vi "Multi_Run_Prog.vi"(0 "Command filename":path, 1 "Setup mode":T9(ring)) -> ()   [LabVIEW 2010]
uses:
  Anemometry Sub Vis/Gen Trav/Traverse_cluster.ctl
  Anemometry Sub Vis/Gen Trav/Spacing.ctl
  Anemometry Sub Vis/Controls/Multi_run_mode.ctl
  Anemometry Sub Vis/Gen Trav/Route mapping/Route_Display_Mode.ctl
  Anemometry Sub Vis/Controls/User_Specific_mode.ctl
  Anemometry Sub Vis/Controls/Multi_Run_Case.ctl
  Anemometry Sub Vis/Gen Trav/Multi_Run_Status.ctl
  Anemometry Sub Vis/Controls/Tunnel_Coordinates.ctl
  Anemometry Sub Vis/Controls/Post_Process.ctl
  ADAM Client/Sub VIs/ADAM Controls/Traverse_Level_State.ctl
  ADAM Client/Sub VIs/ADAM Controls/Tunnel_speed_mode.ctl
  Anemometry Sub Vis/Controls/Overhead.ctl
  ADAM Client/Sub VIs/ADAM Controls/Remember_value_mode.ctl
  Anemometry Sub Vis/Gen Trav/Trav_mode.ctl
  ADAM Client/Sub VIs/ADAM Controls/Client_Source_Status.ctl
  ADAM Client/Sub VIs/ADAM Controls/Update_scan_value.ctl
  Anemometry Sub Vis/File/Setup_Filetype.ctl
  Anemometry Sub Vis/Globals/Meas_global.vi
  Anemometry Sub Vis/Globals/Trav_pos_global.vi
  Anemometry Sub Vis/Globals/Preference_global.vi
  Anemometry Sub Vis/Gen Trav/Route mapping/Route_mapping_global.vi
  Anemometry Sub Vis/Globals/Extra_Commands_Global.vi
  Anemometry Sub Vis/Globals/LDA_meas_global_2.vi
  Anemometry Sub Vis/Globals/LDA_meas_global_1.vi
panel:
  out "Last Row Run":i32
  in  "Stop after Repeats":bool
  in  "Jump Bad Positions":bool
  in  "Work in Tunnel Coordinates?":T1
  out "Current Overhead Factor":dbl format="%.3f"
  out "Estimated Completion time":string
  out "Max Tunnel Speed":dbl format="%.2f"
  out "Pause message":string
  in  "Pause":bool
  out "Non Starter":bool
  out "No of Rows":i32
  out "Status":T2
  in  "Synchronization Start No":i32=1 min=1 max=100
  out "Multi Run Case":T3
  out "Simulate/Run":T4
  in  "Display Mode":T5=enum."Display View on Crash"
  in  "stop":bool
  out "Currently on Row":i32
  in  "Table":T6[](array[typedef]) {"Row Duration (mins)" format="%#.1f"; "Row No" min=0; "Trace Gas Concentration (%)" min=0.0 format="%#.2f"; "Emission Rate (l/min)" format="%#.2f"; "Tunnel Speed" format="%#.2f"; "Start X" format="%#.2f"; "Start Y" format="%#.2f"; "Start Z" format="%#.2f"; "End X" format="%#.2f"; "End Y" format="%#.2f"; "End Z" format="%#.2f"; "Averaging time (min)" min=0.0 format="%#.2f"}
  # "X           Y            Z"
  # "Start"
  # "End"
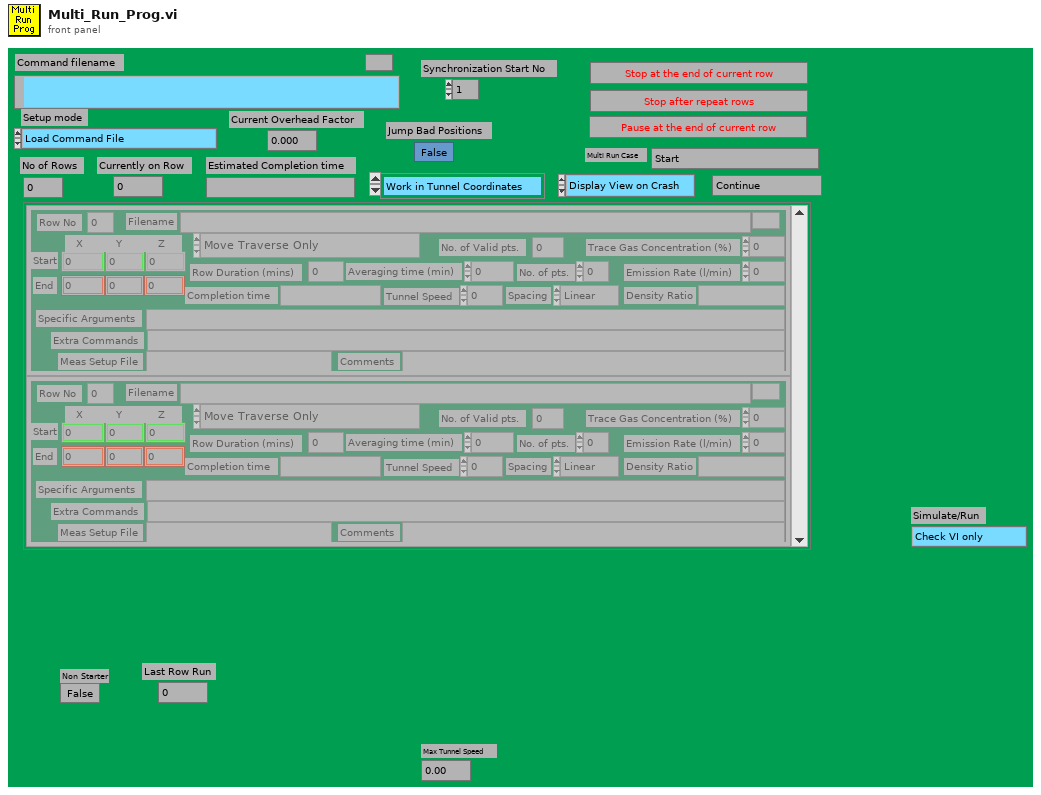
[diagram p1: front panel]
types:
  T1 = typedef "Tunnel_Coordinates.ctl" = enum16{"Work in Tunnel Coordinates", "Work in Model Coordinates"}
  T2 = typedef "Multi_Run_Status.ctl" = enum16{"Continue", "Jump to Next Point", "Jump to Next Row", "Jump To Fall Back", "Terminate Run"}
  T3 = typedef "Multi_Run_Case.ctl" = enum16{"Start", "Load Setup From File", "Has file been edited in Excel?", "Check Max Tunnel Speed", "Pre Check Row", "Check Rows", "Remove blank end rows", "Do results files already exist?", "FFID Bkgnd Measurements?", "First Save Setup file", "Setup Route checking", "Initialise Measurement Prog", "Input Current Position", "Experimental setup control", "Check source flowrates", "Setup for running mode", "Skip Blank Rows", "Which row to execute next", "Evaluate IF Statement", "Perform Measurement Setup", "Set Measurement Conditions", "Execute Row", "Calculate Row TIme", "Update time estimate", "Pause Multi Run Program", "Do Another Row?", "Find Next Fall Back Row", "Shut down source etc", "Email results to users", "Save run efficiency", "Remove Skipped Commands", "Show jumped positions", "Save Setup to File", "End"}
  T4 = typedef "User_Specific_mode.ctl" = enum16{"Check VI only", "Run VI"}
  T5 = typedef "Route_Display_Mode.ctl" = enum16{"Display View Always", "Display View on Crash"}
  T6 = typedef "Traverse_cluster.ctl" = cluster{"Start X":dbl, "Start Y":dbl, "Start Z":dbl, "End X":dbl, "End Y":dbl, "End Z":dbl, "No. of pts.":i32, "Spacing":T7, "Filename":path, "Tunnel Speed":dbl, "Averaging time (min)":dbl, "Extra Commands":string, "Specific Arguments":string, "Emission Rate (l/min)":dbl, "Trace Gas Concentration (%)":dbl, "Density Ratio":string, "Comments":string, "Row No":i32, "Row Type Selector":T8, "Completion time":string, "Row Duration (mins)":dbl, "No. of Valid pts.":i32, "Meas Setup File":string}
  T7 = typedef "Spacing.ctl" = enum16{"Linear", "Log", "Gauss", "Specified", "N/A"}
  T8 = typedef "Multi_run_mode.ctl" = enum16{"Move Traverse Only", "Set Tunnel Speed Only", "Set Source Only", "Set Measurement Conditions", "Single Measurement", "Vertical Profile", "Lateral Profile", "Longitudinal Profile", "Explore Volume", "Multi-Axis Profile", "Auto Calibrate", "Meas Fast FID Bkgnd", "Check Beam Power", "Scanning Valve Measurement", "Run VI Named:", "Set ADAM Ch", "Wait (minutes)", "Send Message", "Synchronize With:", "Fall Back to this Row", "Turn Off Row Repeating", "Blank Row"}
  T9 = enum16{"Load Command File", "Save Command File", "Check Multi Run Prog", "Check Multi Run Prog With Live Moves", "Run Multi Run Prog"}
  T10 = typedef "Post_Process.ctl" = enum16{"Take New Data", "Post Process Raw Data File"}
  T11 = typedef "Traverse_Level_State.ctl" = enum16{"Running", "Complete"}
  T12 = enum32{"existing file", "new file", "new or existing file", "existing dir", "new dir", "new or existing dir", "existing file (use LLBs)", "new file (use LLBs)", "new or existing file (use LLBs)", "new or existing file or directory (use LLBs)"}
  T13 = typedef "Tunnel_speed_mode.ctl" = enum16{"Set Speed", "Set Speed then wait", "Is tunnel speed allowable?"}
  T14 = enum16{"All Channel Names", "Valid Channel Names"}
  T15 = typedef "Overhead.ctl" = enum16{"Update total times", "Read Current Overhead", "Re Scale totals to 3 hrs", "Initialise totals to 3hr"}
  T16 = typedef "Remember_value_mode.ctl" = enum16{"Read only", "Read and Write"}
  T17 = typedef "Trav_mode.ctl" = enum16{"Move traverse", "Read traverse position", "Teach Position"}
  T18 = typedef "Client_Source_Status.ctl" = enum16{"Not Using", "Using", "Must Have"}
  T19 = typedef "Update_scan_value.ctl" = cluster{"Channel Name":string, "New Value":dbl}
  T20 = typedef "Setup_Filetype.ctl" = enum16{"Measurement Setups", "Calibration Setups", "General", "Results File Plotter Setups", "Speed Calib Tweaks"}
  T21 = enum16{"To Traverse Coordinates", "To User Coordinates"}
  T22 = typedef "Status_Cluster.ctl" = cluster{"Status":T2, "Error Type":string, "Error Description":string}
  T23 = typedef "BSA_info_Cluster.ctl" = cluster{"GPIB Address":string, "No of Check Bytes":i32, "Extra Info":string, "COLOUR":u32, "Wavelength (nm)":dbl}
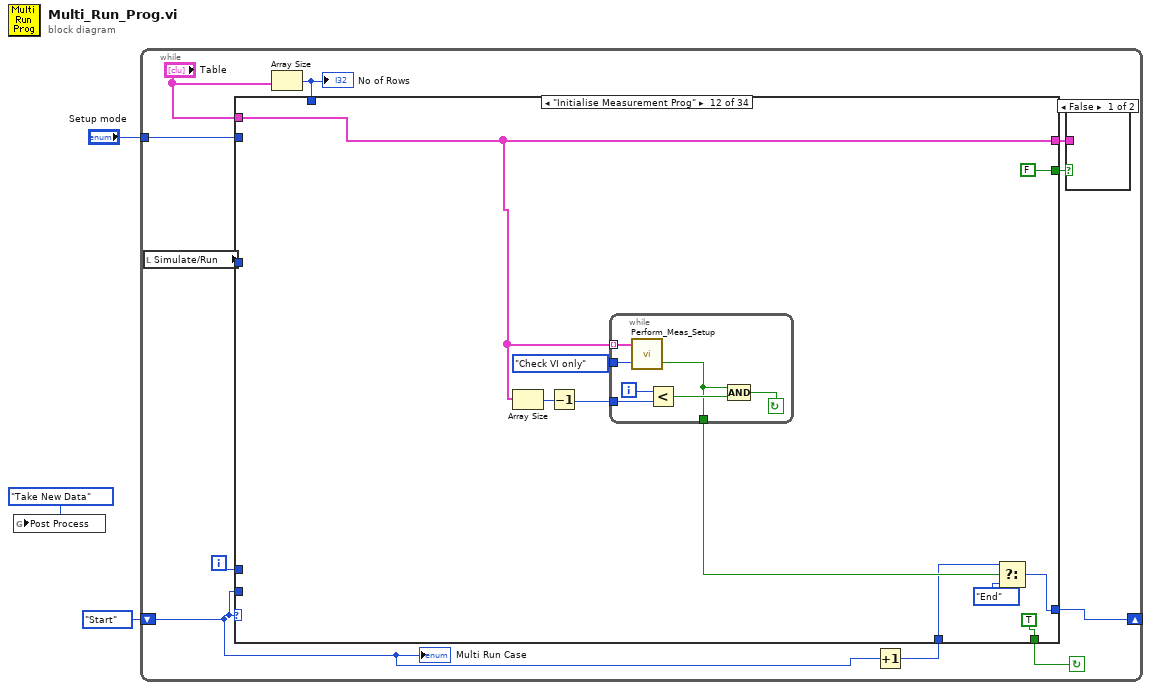
[diagram p0: block diagram]
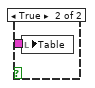
[diagram p2: hidden frame]
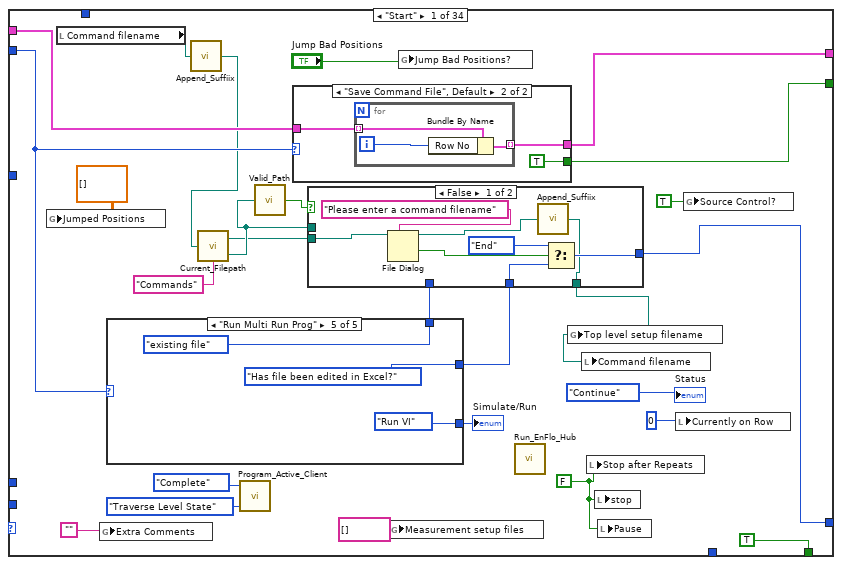
[diagram p3: hidden frame]
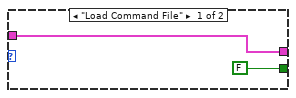
[diagram p4: hidden frame]
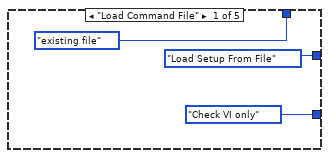
[diagram p6: hidden frame]
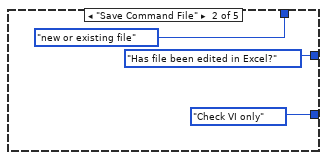
[diagram p7: hidden frame]
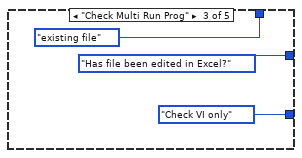
[diagram p8: hidden frame]
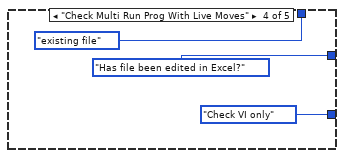
[diagram p9: hidden frame]
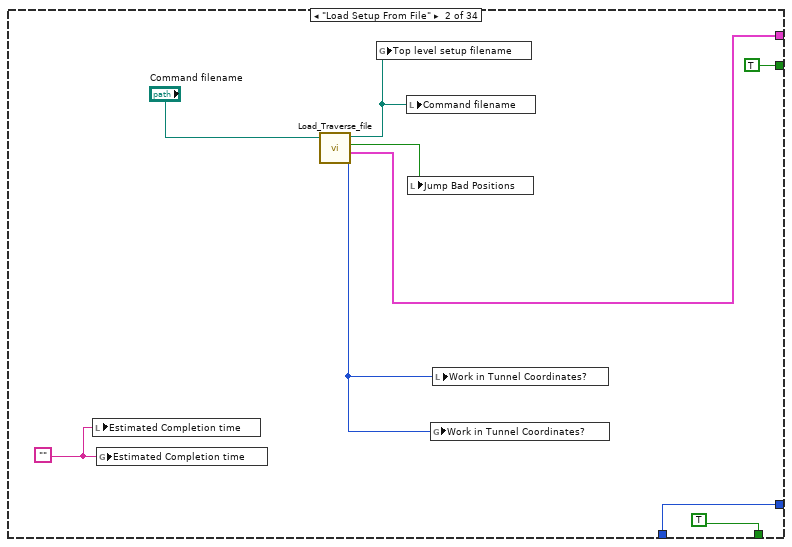
[diagram p10: hidden frame]
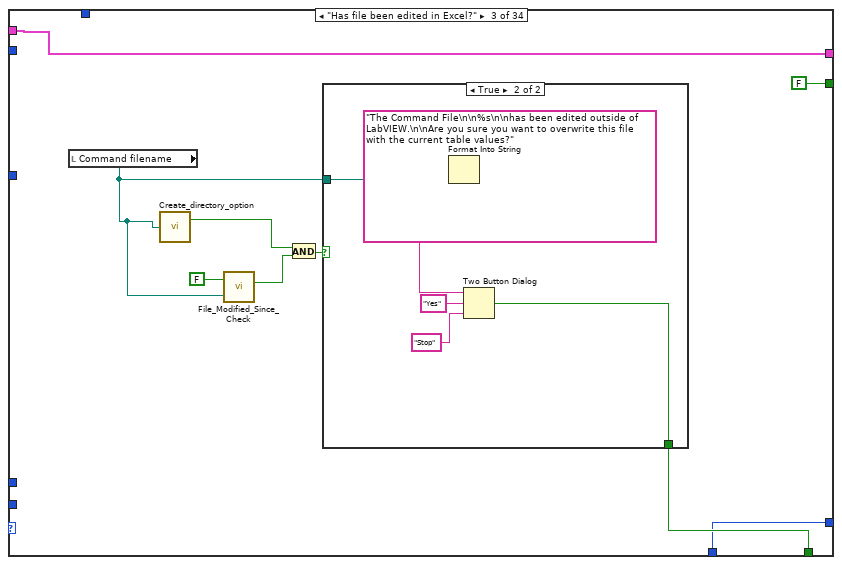
[diagram p11: hidden frame]
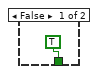
[diagram p12: hidden frame]
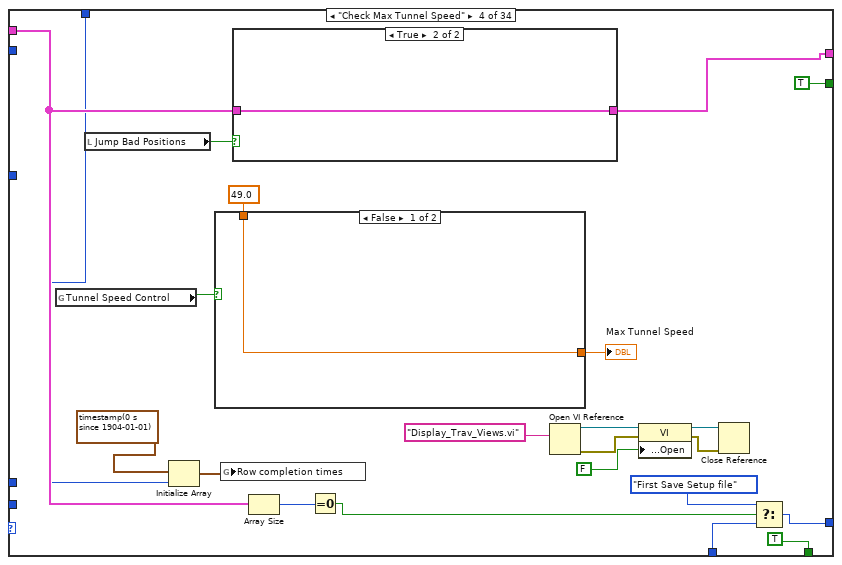
[diagram p13: hidden frame]
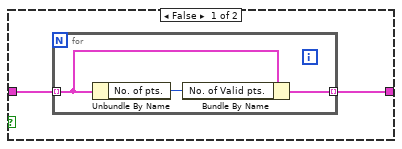
[diagram p14: hidden frame]
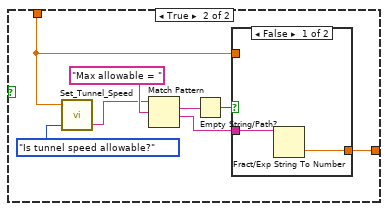
[diagram p15: hidden frame]
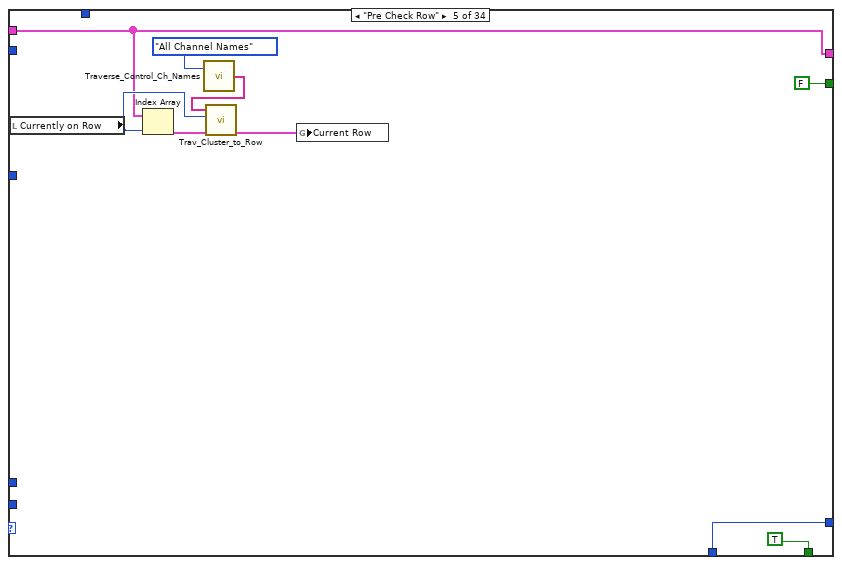
[diagram p17: hidden frame]
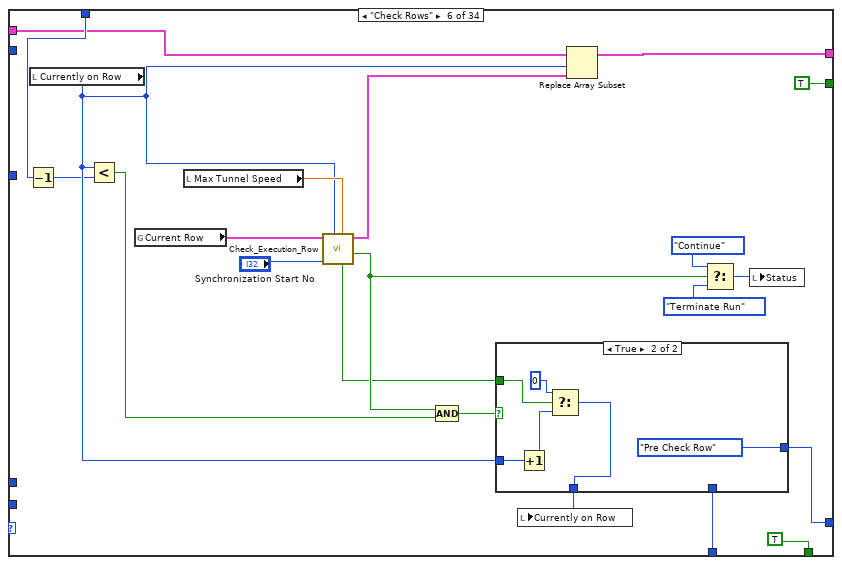
[diagram p18: hidden frame]
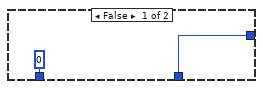
[diagram p19: hidden frame]
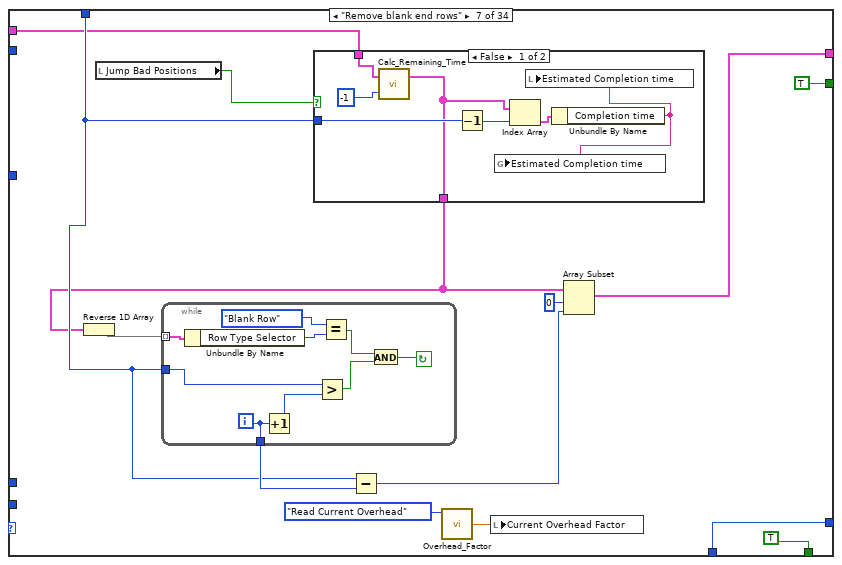
[diagram p20: hidden frame]
diagram:
  n1 = global write "Meas_global.vi" "Post Process"(Post_Process."Take New Data" ("Post Process")) -> ()
  n2 = while {
    shift-left: Multi_Run_Case."Start" ("Multi Run Case") -> [w10]
    shift-right: [w6] -> _
    tunnel: "Setup mode" -> [w13]
    i -> [w11]
    stop <- w14 continue-if-true
    n3 = local read "Simulate/Run"() -> (w7:T4)
    n4 = Array Size(array="Table") -> (size(s)=w5:i32)
    "No of Rows" <- w5
    n5 = Increment(x=w10) -> (x+1=w12:T3)
    n6 = case shown="\"Initialise Measurement Prog\"" w10 {
      tunnel: [TRUE TRUE w87 TRUE TRUE TRUE TRUE TRUE TRUE TRUE TRUE ("Continue?") TRUE ("Continue?") TRUE TRUE TRUE w520 TRUE ("Continue?") TRUE ("Continue?") TRUE TRUE ("Continue?") TRUE TRUE TRUE TRUE TRUE TRUE TRUE TRUE TRUE TRUE TRUE TRUE TRUE FALSE] -> w14
      tunnel: w13 -> [w26 _ _ _ _ _ _ _ _ w395 _ _ _ _ _ _ _ _ _ _ _ _ _ _ _ _ _ _ _ _ _ _ w1245 _]
      tunnel: "Table" -> [w39 _ w84 w114 w142 w154 w179 w210 w368 w397 w416 w456 w469 w497 w507 w523 w575 w619 w735 w786 w798 w889 w925 w957 w998 w1040 w1075 w1105 w1134 w1179 w1184 w1193 w1266 w1329]
      tunnel: w7 -> [_ _ _ _ _ _ _ w209 _ _ _ _ _ w501 w506 w522 _ w617 w732 w783 w796 w888 w923 w954 _ w1049 _ w1096 _ _ _ _ w1256 _]
      tunnel: w10 -> [_ _ _ _ _ _ _ _ _ _ _ _ _ _ _ _ _ _ _ _ _ _ _ _ _ _ _ _ _ _ _ _ _ _]
      tunnel: w12 -> [_ w80 w86 w112 w146 w156 w190 w214 w363 w394 w423 w453 w470 w496 w512 w525 w577 w615 w740 w787 w805 w886 w915 w959 w1001 _ _ w1089 w1136 w1181 w1187 w1201 w1264 w1328]
      tunnel: w11 -> [_ _ _ _ _ _ _ _ _ _ _ _ _ _ _ _ _ _ _ _ _ _ _ _ w999 _ _ _ _ _ _ _ _ _]
      tunnel: [w37 w80 w86 w111 w146 w155 w190 w214 w363 w390 w423 w452 w470 w496 w509 w525 w577 w616 w739 w787 w806 w886 w915 w959 w1002 w1050 w1072 w1100 w1136 w1181 w1187 w1201 w1264 w1328] -> w6
      tunnel: [w25 TRUE FALSE ("Rows Added ?") TRUE ("Rows Added ?") FALSE TRUE TRUE FALSE FALSE TRUE FALSE FALSE FALSE FALSE FALSE TRUE FALSE ("Rows Added ?") FALSE ("Rows Added ?") FALSE FALSE ("Rows Added ?") FALSE FALSE FALSE TRUE ("Rows Added ?") FALSE FALSE FALSE FALSE FALSE FALSE TRUE TRUE TRUE FALSE] -> w8
      tunnel: w5 -> [_ _ _ w106 _ w160 w181 _ _ _ _ _ _ _ _ _ w578 w618 _ _ _ _ _ w953 _ w1035 _ _ _ _ _ _ _ _]
      tunnel: [w38 w81 w84 w116 w142 w163 w185 w210 w368 w398 w416 w456 w469 w497 w507 w521 w575 w620 w735 w786 w798 w889 w925 w956 w998 w1040 w1075 w1105 w1134 w1179 w1183 w1193 w1265 w1329] -> w4
      frame "Start" {
        w23 = FALSE ("Measurment setup Found?")
        n7 = global write "Trav_pos_global.vi" "Jumped Positions"(dbl[][] [] ("Jumped Positions")) -> ()
        n8 = local read "Command filename"() -> (w29:path)
        n9 = global write "Meas_global.vi" "Extra Comments"("") -> ()
        n10 = case shown="\"Run Multi Run Prog\"" w26 {
          tunnel: [User_Specific_mode."Check VI only" ("Simulate/Run") User_Specific_mode."Check VI only" ("Simulate/Run") User_Specific_mode."Check VI only" ("Simulate/Run") User_Specific_mode."Check VI only" ("Simulate/Run") User_Specific_mode."Run VI" ("Simulate/Run")] -> w40
          tunnel: [Multi_Run_Case."Load Setup From File" ("Multi Run Case") Multi_Run_Case."Has file been edited in Excel?" ("Multi Run Case") Multi_Run_Case."Has file been edited in Excel?" ("Multi Run Case") Multi_Run_Case."Has file been edited in Excel?" ("Multi Run Case") Multi_Run_Case."Has file been edited in Excel?" ("Multi Run Case")] -> w36
          tunnel: [T12."existing file" ("select mode (2)") T12."new or existing file" ("select mode (2)") T12."existing file" ("select mode (2)") T12."existing file" ("select mode (2)") T12."existing file" ("select mode (2)")] -> w24
          frame "Load Command File" {
          }
          frame "Save Command File" {
          }
          frame "Check Multi Run Prog" {
          }
          frame "Check Multi Run Prog With Live Moves" {
          }
          frame "Run Multi Run Prog" {
          }
        }
        "Simulate/Run" <- w40
        n11 = call "Append_Suffiix.vi"("Results file"=w29) -> ("appended path"=w18:path)
        n12 = call "Current_Filepath.vi"("Filename in"=w18, "Data Type"="Commands") -> ("Filename Out"=w17:path, "Directory"=w16:path)
        n13 = call "Program_Active_Client.vi"("Mode"=enum16{"Program Active", "Traverse Level State"}."Traverse Level State", "Traverse level State"=Traverse_Level_State."Complete") -> ()  [unwired: 1 in, 3 out]
        n14 = call "Valid_Path.vi"("Filename"=w17) -> ("Valid Path?"=w27:bool)
        n15 = case shown="\"Save Command File\", Default" w26 {
          tunnel: w39 -> [w43 w46]
          tunnel: [w43 w45] -> w38
          tunnel: [FALSE TRUE] -> w25
          frame "Load Command File" {
          }
          frame "Save Command File", Default {
            n16 = for {
              tunnel: w46 -> [w49] mode=indexing
              tunnel: [w48] -> w45 mode=indexing
              i -> [w47]
              n17 = Bundle By Name(cluster=w49, "Row No"=w47) -> (w48:T6)
            }
          }
        }
        n18 = case shown="False" w27 {
          tunnel: [w55 w59] -> w37
          tunnel: w36 -> [w56 w59]
          tunnel: w17 -> [_ w58]
          tunnel: [w54 w58] -> w28
          tunnel: w24 -> [_ _]
          tunnel: w16 -> [w50 _]
          frame False {
            n19 = File Dialog(7:"Please enter a command filename" ("prompt"), 11:w50) -> (1:w52:bool, 3:w53:path)  [unwired: 1 in, 6 out]
            n20 = call "Append_Suffiix.vi"("Results file"=w53) -> ("appended path"=w54:path)
            n21 = Select(t=Multi_Run_Case."End" ("Multi Run Case"), s=w52, f=w56) -> (s? t:f=w55:T3)
          }
          frame True {
          }
        }
        n22 = global write "Trav_pos_global.vi" "Measurement setup files"(string[] [] ("Measurement setup files")) -> ()
        n23 = global write "Trav_pos_global.vi" "Jump Bad Positions?"("Jump Bad Positions") -> ()
        n24 = call "Run_EnFlo_Hub.vi"() -> ()  [unwired: 8 out]
        n25 = global write "Trav_pos_global.vi" "Top level setup filename"(w28) -> ()
        n26 = local write "Command filename"(w28) -> ()
        n27 = local write "Stop after Repeats"(w23) -> ()
        n28 = local write "stop"(w23) -> ()
        n29 = local write "Pause"(w23) -> ()
        n30 = local write "Currently on Row"(0 ("Currently on Row")) -> ()
        n31 = global write "Trav_pos_global.vi" "Source Control?"(TRUE ("Source Control?")) -> ()
        "Status" <- Multi_Run_Status."Continue" ("Status")
      }
      frame "Load Setup From File" {
        w76 = ""
        n32 = local write "Estimated Completion time"(w76) -> ()
        n33 = global write "Trav_pos_global.vi" "Estimated Completion time"(w76) -> ()
        n34 = call "Load_Traverse_file.vi"("Setup filename"="Command filename") -> ("Setup filename Out"=w78:path, "Jump Bad Positions"=w75:bool, "Table"=w81:T6[], "Work in Tunnel Coordinates?"=w77:T1)  [unwired: 2 out]
        n35 = global write "Trav_pos_global.vi" "Top level setup filename"(w78) -> ()
        n36 = local write "Command filename"(w78) -> ()
        n37 = local write "Jump Bad Positions"(w75) -> ()
        n38 = global write "Trav_pos_global.vi" "Work in Tunnel Coordinates?"(w77) -> ()
        n39 = local write "Work in Tunnel Coordinates?"(w77) -> ()
      }
      frame "Has file been edited in Excel?" {
        n40 = local read "Command filename"() -> (w88:path)
        n41 = call "Create_directory_option.vi"("Filename"=w88) -> ("Path is to existing File"=w91:bool)  [unwired: 1 out]
        n42 = call "File_Modified_Since_Check.vi"("Pathname"=w88, "Just Modified?"=FALSE) -> ("Modified?"=w90:bool)
        n43 = And(x=w91, y=w90) -> (x .and. y?=w92:bool)
        n44 = case shown="True" w92 {
          tunnel: w88 -> [_ w99]
          tunnel: [TRUE ("T button?") w94] -> w87
          frame False {
          }
          frame True {
            n45 = Format Into String(format string="The Command File\n\n%s\n\nhas been edited outside of LabVIEW.\n\nAre you sure you want to overwrite this file  with the current table values?" ("Format String"), w99) -> (resulting string=w97:string)  [unwired: 2 in, 1 out]
            n46 = Two Button Dialog(message=w97, 1:"Stop" ("F button name (\"Cancel\")"), 2:"Yes" ("T button name (\"OK\")")) -> (T button?=w94:bool)
          }
        }
      }
      frame "Check Max Tunnel Speed" {
        n47 = global read "Preference_global.vi" "Tunnel Speed Control"() -> (w117:bool)
        n48 = local read "Jump Bad Positions"() -> (w115:bool)
        n49 = Initialize Array(timestamp(0 s since 1904-01-01) ("seconds since 1Jan1904"), w106) -> (w107:timestamp[])
        n50 = case shown="False" w117 {
          tunnel: 49.0 ("Tunnel Velocity m/s") -> [w128 w129]
          tunnel: [w128 w131] -> w119
          frame False {
          }
          frame True {
            n51 = call "Set_Tunnel_Speed.vi"("Mode"=Tunnel_speed_mode."Is tunnel speed allowable?", "Tunnel Velocity m/s"=w129) -> ("Error String"=w134:string)  [unwired: 1 in, 2 out]
            n52 = Match Pattern(string=w134, regular expression="Max allowable = ") -> (match substring=w133:string, after substring=w130:string)  [unwired: 3 out]
            n53 = Empty String/Path?(string/path=w133) -> (empty?=w132:bool)
            n54 = case shown="False" w132 {
              tunnel: [w137 w139] -> w131
              tunnel: w129 -> [_ w139]
              tunnel: w130 -> [w138 _]
              frame False {
                n55 = Fract/Exp String To Number(string=w138) -> (number=w137:dbl)  [unwired: 4 out]
              }
              frame True {
              }
            }
          }
        }
        "Max Tunnel Speed" <- w119
        n56 = global write "Trav_pos_global.vi" "Row completion times"(w107) -> ()
        n57 = case shown="True" w115 {
          tunnel: w114 -> [w123 w127]
          tunnel: [w122 w127] -> w116
          frame False {
            n58 = for {
              tunnel: w123 -> [w125] mode=indexing
              tunnel: [w124] -> w122 mode=indexing
              n59 = Unbundle By Name(w125) -> ("No. of pts."=w126:i32)
              n60 = Bundle By Name(cluster=w125, "No. of Valid pts."=w126) -> (w124:T6)
            }
          }
          frame True {
          }
        }
        n61 = Array Size(array=w114) -> (size(s)=w113:i32)
        n62 = Equal To 0?(x=w113) -> (x = 0?=w110:bool)
        n63 = Open VI Reference(vi path="Display_Trav_Views.vi" ("VI path")) -> (vi reference=w105:refnum<vi>, error out=w104:errorcluster)  [unwired: 1 in, 4 out]
        n64 = property class="VI"(reference=w105, error in=w104, "Front Panel Window:Open"=FALSE) -> (reference out=w102:refnum<vi>, error out=w101:errorcluster)
        n65 = Close Reference(reference=w102, error in (no error)=w101) -> ()  [unwired: 1 out]
        n66 = Select(t=Multi_Run_Case."First Save Setup file" ("Multi Run Case"), s=w110, f=w112) -> (s? t:f=w111:T3)
      }
      frame "Pre Check Row" {
        n67 = local read "Currently on Row"() -> (w143:i32)
        n68 = Index Array(array=w142, index=w143) -> (element=w144:T6)
        n69 = call "Traverse_Control_Ch_Names.vi"("Mode"=T14."All Channel Names") -> ("Channel names"=w140:string[])  [unwired: 1 in]
        n70 = call "Trav_Cluster_to_Row.vi"("Traverse line in"=w144, "Row Number"=w143, "Channel names"=w140) -> ("Traverse line Out"=w145:T6)  [unwired: 4 out]
        n71 = global write "Trav_pos_global.vi" "Current Row"(w145) -> ()
      }
      frame "Check Rows" {
        n72 = Decrement(x=w160) -> (x-1=w150:i32)
        n73 = local read "Currently on Row"() -> (w151:i32)
        n74 = Less?(x=w151, y=w150) -> (x < y?=w159:bool)
        n75 = global read "Trav_pos_global.vi" "Current Row"() -> (w152:T6)
        n76 = local read "Max Tunnel Speed"() -> (w162:dbl)
        n77 = call "Check_Execution_Row.vi"("Execution Row"=w152, "Synchronization Start No"="Synchronization Start No", "Row Index"=w151, "Max Tunnel Speed"=w162) -> ("Editted Row"=w149:bool, "Execution Row Out"=w153:T6, "Continue?"=w161:bool)  [unwired: 1 in, 3 out]
        n78 = Compound Arithmetic op=AND(w161, w159) -> (w158:bool)
        n79 = case shown="True" w158 {
          tunnel: [0 w173] -> w157
          tunnel: w151 -> [_ w177]
          tunnel: w156 -> [w171 _]
          tunnel: [w171 Multi_Run_Case."Pre Check Row" ("Multi Run Case")] -> w155
          tunnel: w149 -> [_ w175]
          frame False {
          }
          frame True {
            n80 = Increment(x=w177) -> (x+1=w174:i32)
            n81 = Select(t=0, s=w175, f=w174) -> (s? t:f=w173:i32)
          }
        }
        n82 = local write "Currently on Row"(w157) -> ()
        n83 = Replace Array Subset(array=w154, new element=w153, index=w151) -> (w163:T6[])
        n84 = Select(t=Multi_Run_Status."Continue" ("Status"), s=w161, f=Multi_Run_Status."Terminate Run" ("Status")) -> (s? t:f=w167:T2)
        n85 = local write "Status"(w167) -> ()
      }
      frame "Remove blank end rows" {
        n86 = local read "Jump Bad Positions"() -> (w178:bool)
        n87 = case shown="False" w178 {
          tunnel: w181 -> [w196 _]
          tunnel: w179 -> [w195 w199]
          tunnel: [w193 w199] -> w180
          frame False {
            n88 = call "Calc_Remaining_Time.vi"("Currently on Row"=-1 ("Start Index"), "Table In"=w195) -> ("Table Out"=w193:T6[])  [unwired: 1 out]
            n89 = Decrement(x=w196) -> (x-1=w198:i32)
            n90 = Index Array(array=w193, index=w198) -> (element=w197:T6)
            n91 = Unbundle By Name(w197) -> ("Completion time"=w192:string)
            n92 = global write "Trav_pos_global.vi" "Estimated Completion time"(w192) -> ()
            n93 = local write "Estimated Completion time"(w192) -> ()
          }
          frame True {
          }
        }
        n94 = Reverse 1D Array(array=w180) -> (reversed array=w189:T6[])
        n95 = while {
          tunnel: [w200] -> w187
          tunnel: w181 -> [w204]
          tunnel: w189 -> [w208] mode=indexing
          i -> [w200]
          stop <- w201 continue-if-true
          n96 = Unbundle By Name(w208) -> ("Row Type Selector"=w206:T8)
          n97 = Increment(x=w200) -> (x+1=w205:i32)
          n98 = Greater?(x=w204, y=w205) -> (0:w203:bool)
          n99 = Equal?(x=Multi_run_mode."Blank Row" ("Row Type Selector"), y=w206) -> (x = y?=w202:bool)
          n100 = And(x=w202, y=w203) -> (x .and. y?=w201:bool)
        }
        n101 = Subtract(x=w181, y=w187) -> (x-y=w186:i32)
        n102 = call "Overhead_Factor.vi"("Mode"=Overhead."Read Current Overhead") -> ("Current Overhead Factor"=w182:dbl)  [unwired: 3 in]
        n103 = local write "Current Overhead Factor"(w182) -> ()
        n104 = Array Subset(array=w180, index=0 ("Array Index"), length=w186) -> (w185:T6[])
      }
      frame "Do results files already exist?" {
        n105 = for {
          tunnel: w210 -> [w226] mode=indexing
          tunnel: [w224] -> w216 mode=indexing
          shift-right: [w220] -> _
          shift-left: path[] [] -> [w221]
          tunnel: w209 -> [w218]
          n106 = Unbundle By Name(w226) -> ("Specific Arguments"=w217:string, "Emission Rate (l/min)"=w225:dbl, "Row Type Selector"=w223:T8, "Filename"=w222:path)
          n107 = while {
            shift-left: w221 -> [w234]
            shift-right: [w233] -> w220
            tunnel: w222 -> [w235]
            tunnel: w223 -> [w239]
            shift-left: 0 -> [w240]
            shift-right: [w236] -> _
            tunnel: w218 -> [w230]
            shift-right: [w229] -> _
            shift-left: _ -> [w228]
            tunnel: w217 -> [w227]
            stop <- w238 continue-if-true
            n108 = Increment(x=w240) -> (x+1=w237:i32)
            n109 = case shown="0, Default" w240 {
              tunnel: w239 -> [w249 _ _ _ _ _ _ _ _ _ _ _]
              tunnel: [w244 w269 w274 w281 w286 TRUE ("exists?") TRUE ("exists?") FALSE ("exists?") FALSE ("exists?") TRUE ("true") w343 w356] -> w238
              tunnel: w237 -> [w251 w272 w277 w280 w287 w292 w303 w314 w325 w329 w341 _]
              tunnel: [w251 w272 w277 w280 w287 w290 w302 w314 w325 w330 w341 w355] -> w236
              tunnel: [w250 w271 w276 w279 w284 w300 w311 w316 w318 w327 w345 w361] -> w233
              tunnel: w234 -> [w250 w271 w276 w279 w285 w300 w311 w316 w318 w327 w345 w361]
              tunnel: w235 -> [w243 _ _ _ _ _ _ _ _ _ _ _]
              tunnel: 7 -> [_ _ _ _ _ _ _ _ _ w328 _ w355]
              tunnel: 9 -> [_ _ _ _ _ w291 _ _ _ _ _ _]
              tunnel: w230 -> [_ _ _ _ _ _ _ _ _ _ w344 _]
              tunnel: [w242 w268 w273 w278 w283 w288 w301 w312 w317 w326 w342 w354] -> w229
              tunnel: w228 -> [_ w268 w273 w278 w283 w288 w301 w312 w317 w326 w342 w354]
              tunnel: w227 -> [w241 _ _ _ _ _ _ _ _ _ _ _]
              frame 0, Default {
                n110 = case shown="\"Run VI Named:\"" w249 {
                  tunnel: [TRUE w259 FALSE FALSE] -> w246
                  tunnel: w243 -> [w252 w258 w264 w266]
                  tunnel: w241 -> [_ w256 _ _]
                  tunnel: [w252 w258 w264 w266] -> w242
                  frame "Move Traverse Only", Default {
                  }
                  frame "Run VI Named:" {
                    n111 = Match Pattern(string=w256, regular expression=";") -> (before substring=w255:string)  [unwired: 4 out]
                    n112 = call <vilib>:"Trim Whitespace.vi"("string"=w255) -> ("trimmed string"=w254:string)  [unwired: 1 in]
                    n113 = Equal?(x=w254, y="Pressure_Tapped_Cube.vi") -> (x = y?=w260:bool)
                    n114 = Equal?(x=w254, y="Take_Data_on_the_Move.vi") -> (x = y?=w261:bool)
                    n115 = Or(x=w260, y=w261) -> (x .or. y?=w259:bool)
                  }
                  frame "Auto Calibrate" {
                  }
                  frame "Send Message" {
                  }
                }
                n116 = local read "Status"() -> (w247:T2)
                n117 = Not Equal?(x=Multi_Run_Status."Terminate Run" ("Status"), y=w247) -> (x != y?=w245:bool)
                n118 = And(x=w246, y=w245) -> (x .and. y?=w244:bool)
              }
              frame 1 {
                n119 = Not Equal?(x=path "", y=w268) -> (x != y?=w269:bool)
              }
              frame 2 {
                n120 = Not Equal?(x=w273, y=path "") -> (x != y?=w274:bool)
              }
              frame 3 {
                n121 = Search 1D Array(1D array=w279, element=w278) -> (index of element=w282:i32)  [unwired: 1 out]
                n122 = Less Than 0?(x=w282) -> (x < 0?=w281:bool)
              }
              frame 4 {
                n123 = Build Array (concatenate)(w285, w283) -> (w284:path[])
                n124 = call "Does_file_exist_(simple).vi"("Pathname"=w283) -> ("exists?"=w286:bool)
              }
              frame 5 {
                n125 = Path To String(path=w288) -> (string=w299:string)
                n126 = global read "Meas_global.vi" "Start Time of experiment"() -> (w294:dbl)
                n127 = Concatenate Strings(w299, "Append" ("Substring")) -> (w297:string)
                n128 = call "Remember_value.vi"("Mode"=Remember_value_mode."Read only", "Ch name"=w297) -> ("Output Value"=w295:dbl)  [unwired: 1 in]
                n129 = Not Equal?(x=w294, y=w295) -> (x != y?=w293:bool)
                n130 = Select(t=w292, s=w293, f=w291) -> (s? t:f=w290:i32)
              }
              frame 6 {
                n131 = Increment(x=w303) -> (x+1=w304:i32)
                n132 = Format Into String(format string="The results filename \"%s\" already exists.\nDo you wish to append to this file during the run?" ("Format String"), w301) -> (resulting string=w308:string)  [unwired: 2 in, 1 out]
                n133 = Two Button Dialog(message=w308, 1:"Abort Run" ("F button name (\"Cancel\")"), 2:"Append" ("T button name (\"OK\")")) -> (T button?=w305:bool)
                n134 = Select(t=w304, s=w305, f=w303) -> (s? t:f=w302:i32)
              }
              frame 7 {
                n135 = local write "Status"(Multi_Run_Status."Terminate Run" ("Status")) -> ()
              }
              frame 8 {
                n136 = Path To String(path=w317) -> (string=w324:string)
                n137 = Concatenate Strings(w324, "Append" ("Substring")) -> (w322:string)
                n138 = global read "Meas_global.vi" "Start Time of experiment"() -> (w319:dbl)
                n139 = call "Remember_value.vi"("Mode"=Remember_value_mode."Read and Write", "Input Value"=w319, "Ch name"=w322) -> ()  [unwired: 1 out]
              }
              frame 9 {
                n140 = call "Read_File_Simple.vi"("Filename"=w326) -> ("string"=w333:string)  [unwired: 2 in, 7 out]
                n141 = call "Is_it_a_Results_File.vi"("character string"=w333) -> ("Results File?"=w332:bool)  [unwired: 2 out]
                n142 = case shown="True" w332 {
                  tunnel: w326 -> [w336 _]
                  tunnel: [w334 w340] -> w330
                  tunnel: w329 -> [_ w340]
                  tunnel: w328 -> [w334 _]
                  frame False {
                    n143 = Path To String(path=w336) -> (string=w338:string)
                    n144 = Format Into String(format string="The File %s is not in the correct Results file format.\nCheck that it is tab delimited rather than excel format, or choose another file." ("Format String"), w338) -> (resulting string=w335:string)  [unwired: 2 in, 1 out]
                    n145 = One Button Dialog(message=w335, button name ("OK")="Stop") -> ()  [unwired: 1 out]
                  }
                  frame True {
                  }
                }
              }
              frame 10 {
                n146 = case shown="\"Check VI only\", Default" w344 {
                  tunnel: w342 -> [_ w353]
                  tunnel: [FALSE ("exists?") w347] -> w343
                  frame "Check VI only", Default {
                  }
                  frame "Run VI" {
                    n147 = call "Open_File_for_write.vi"("append to file? (new file:F)"=TRUE, "file path"=w353) -> ("error out"=w351:errorcluster, "refnum"=w352:refnum<file>)  [unwired: 1 in, 7 out]
                    n148 = Unbundle By Name(w351) -> ("code"=w350:i32)
                    n149 = Close File(refnum=w352, error in=w351) -> ()  [unwired: 2 out]
                    n150 = Equal?(x=10 ("code"), y=w350) -> (x = y?=w347:bool)
                  }
                }
              }
              frame 11 {
                n151 = Path To String(path=w354) -> (string=w359:string)
                n152 = Format Into String(format string="The File %s is already open in another application." ("Format String"), w359) -> (resulting string=w358:string)  [unwired: 2 in, 1 out]
                n153 = One Button Dialog(message=w358, button name ("OK")="Stop") -> (true=w356:bool)
              }
            }
          }
          n154 = Greater Than 0?(x=w225) -> (x > 0?=w224:bool)
        }
        n155 = Or Array Elements(Boolean array=w216) -> (logical OR=w212:bool)
        n156 = global write "Trav_pos_global.vi" "Source Control?"(w212) -> ()
      }
      frame "FFID Bkgnd Measurements?" {
        n157 = for {
          tunnel: w368 -> [w384] mode=indexing
          tunnel: [w372] -> w367 mode=indexing
          tunnel: [w373] -> w366 mode=indexing
          n158 = Unbundle By Name(w384) -> ("Row Type Selector"=w378:T8, "Specific Arguments"=w380:string)
          n159 = call "Get_array_values_fr_String.vi"("String Value"=w380) -> ("String array"=w381:string[])  [unwired: 1 out]
          n160 = Index Array(array=w381, index=0 ("Index")) -> (element=w377:string)
          n161 = Equal?(x=Multi_run_mode."Auto Calibrate" ("Row Type Selector"), y=w378) -> (x = y?=w374:bool)
          n162 = Equal?(x=w377, y="Concentration") -> (x = y?=w375:bool)
          n163 = Equal?(x=Multi_run_mode."Meas Fast FID Bkgnd" ("Row Type Selector"), y=w378) -> (x = y?=w372:bool)
          n164 = And(x=w374, y=w375) -> (x .and. y?=w373:bool)
        }
        n165 = Or Array Elements(Boolean array=w367) -> (logical OR=w364:bool)
        n166 = Or Array Elements(Boolean array=w366) -> (logical OR=w365:bool)
        n167 = Compound Arithmetic op=AND(invert w364, w365) -> (w362:bool)
        n168 = case shown="True" w362 {
          frame False {
          }
          frame True {
            n169 = One Button Dialog(message="This run automatically calibrates the Fast FID but does not have a Meas Fast FID Bkgnd row" ("format string")) -> ()  [unwired: 2 out]
          }
        }
      }
      frame "First Save Setup file" {
        w385 = -1 ("Currently on Row")
        n170 = case shown="\"Check Multi Run Prog\"" w395 {
          tunnel: [w402 w404 w406 Multi_Run_Case."End" ("Multi Run Case") Multi_Run_Case."End" ("Multi Run Case")] -> w389
          tunnel: w394 -> [w402 w404 w406 _ _]
          tunnel: [w403 w405 w407 w408 w410] -> w388
          frame "Run Multi Run Prog" {
            w403 = FALSE  # Live Traverse Preview?
          }
          frame "Check Multi Run Prog With Live Moves" {
            w405 = TRUE  # Live Traverse Preview?
          }
          frame "Check Multi Run Prog" {
            w407 = FALSE  # Live Traverse Preview?
          }
          frame "Load Command File" {
            w408 = FALSE  # Live Traverse Preview?
          }
          frame "Save Command File" {
            w410 = FALSE  # Live Traverse Preview?
          }
        }
        n171 = local read "Command filename"() -> (w396:path)
        n172 = global write "Trav_pos_global.vi" "Work in Tunnel Coordinates?"("Work in Tunnel Coordinates?") -> ()
        n173 = local write "Currently on Row"(w385) -> ()
        n174 = local write "Last Row Run"(w385) -> ()
        n175 = local read "Jump Bad Positions"() -> (w386:bool)
        n176 = call "Save_Trav_setup.vi"("Work in Tunnel Coordinates?"="Work in Tunnel Coordinates?", "Trav Table"=w397, "Jump Bad Positions"=w386, "Setup filename"=w396) -> ("Trav Table Out"=w398:T6[])  [unwired: 1 out]
        n177 = global write "Meas_global.vi" "Extra Comments"("") -> ()
        n178 = global write "Trav_pos_global.vi" "Live Traverse Preview?"(w388) -> ()
        n179 = local read "Status"() -> (w391:T2)
        n180 = case shown="\"Continue\"" w391 {
          tunnel: [w400 Multi_Run_Case."End" ("Multi Run Case")] -> w390
          tunnel: w389 -> [w400 _]
          frame "Continue" {
          }
          frame "Jump to Next Point", Default {
          }
        }
      }
      frame "Setup Route checking" {
        n181 = global read "Preference_global.vi" "Rig Setup"() -> (w418:string)
        n182 = Match Pattern(string=w418, regular expression="-") -> (before substring=w417:string)  [unwired: 4 out]
        n183 = for {
          tunnel: w416 -> [w437] mode=indexing
          shift-right: [w428] -> w414
          shift-left: string[] [] -> [w429]
          n184 = Unbundle By Name(w437) -> ("Extra Commands"=w430:string, "Start X"=w434:dbl, "Start Y"=w433:dbl, "Start Z"=w432:dbl)
          n185 = Build Array(w434, w433, w432) -> (w435:dbl[])
          n186 = Not A Number/Path/Refnum?(number/path/refnum=w435) -> (NaN/Path/Refnum?=w436:bool[])
          n187 = Or Array Elements(Boolean array=w436) -> (logical OR=w431:bool)
          n188 = case shown="False" w431 {
            tunnel: w430 -> [w441 _]
            tunnel: w429 -> [w440 w442]
            tunnel: [w439 w442] -> w428
            frame False {
              n189 = call "Which_Trav_Setup.vi"("Extra Command String"=w441) -> ("Traverse Setup"=w438:string)
              n190 = Build Array (concatenate)(w440, w438) -> (w439:string[])
            }
            frame True {
            }
          }
        }
        n191 = case shown="\"EnFlo_Tunnel\"" w417 {
          frame "No Match", Default {
          }
          frame "EnFlo_Tunnel" {
            w443 = 0.0 ("element")
            n192 = Build Array("EnFlo_Tunnel:Obstacle:Orientation") -> (w450:string[])
            n193 = call "Get_Current_Scan_client.vi"("ADAM Ch Names"=w450) -> ("Numerical Values"=w449:dbl[])  [unwired: 3 out]
            n194 = Index Array(array=w449, index=0) -> (element=w444:dbl)
            n195 = global write "Trav_pos_global.vi" "Model Rotation (deg)"(w444) -> ()
            n196 = Build Array(w444, w443, w443) -> (w445:dbl[])
            n197 = call "Read-Write_Check_Pos.vi"("Position input"=w445, "Mode"=enum16{"Read", "Write"}."Write", "Traverse Name"="EnFlo_Turntable") -> ()  [unwired: 1 out]
          }
        }
        n198 = global write "Route_mapping_global.vi" "Display Mode"("Display Mode") -> ()
        n199 = global read "Trav_pos_global.vi" "Work in Tunnel Coordinates?"() -> (w412:T1)
        n200 = call "Analyse_string_array.vi"("String array"=w414) -> ("Unique strings"=w413:string[])  [unwired: 2 out]
        n201 = for {
          tunnel: w413 -> [w427] mode=indexing
          tunnel: w412 -> [w424]
          n202 = call "3D_Traverse_move.vi"("Mode"=Trav_mode."Read traverse position", "Work in Tunnel Coordinates"=w424, "Simulate/Run"=User_Specific_mode."Run VI", "Traverse name"=w427) -> ()  [unwired: 5 in, 7 out]
        }
      }
      frame "Initialise Measurement Prog" {
        n203 = Array Size(array=w456) -> (size(s)=w457:i32)
        n204 = Decrement(x=w457) -> (x-1=w458:i32)
        n205 = while {
          tunnel: [w462] -> w454
          tunnel: User_Specific_mode."Check VI only" ("Simulate/Run") -> [w463]
          tunnel: w458 -> [w466]
          tunnel: w456 -> [w468] mode=indexing
          i -> [w467]
          stop <- w464 continue-if-true
          n206 = call "Perform_Meas_Setup.vi"("Simulate/Run"=w463, "Traverse line"=w468) -> ("Continue?"=w462:bool)  [unwired: 1 out]
          n207 = Less?(x=w467, y=w466) -> (x < y?=w465:bool)
          n208 = Compound Arithmetic op=AND(w462, w465) -> (w464:bool)
        }
        n209 = Select(t=w453, s=w454, f=Multi_Run_Case."End" ("Multi Run Case")) -> (s? t:f=w452:T3)
      }
      frame "Input Current Position" {
        n210 = disable-structure shown="Disabled" {
          disable-tunnel: w469 -> [w477 _]
          frame Disabled {
            n211 = global read "Trav_pos_global.vi" "Default Traverse Setup"() -> (w475:string)
            n212 = Build Array(w475) -> (w474:string[])
            n213 = global read "Extra_Commands_Global.vi" "!Traverse Setup"() -> (w476:string)
            n214 = for {
              tunnel: w477 -> [w490] mode=indexing
              tunnel: w476 -> [w488]
              shift-right: [w486] -> w473
              shift-left: w474 -> [w487]
              n215 = Unbundle By Name(w490) -> ("Extra Commands"=w489:string)
              n216 = call "Extra_Commands.vi"("String to Search"=w489, "Command"=w488) -> ("String Value"=w485:string, "Command Found"=w483:bool)  [unwired: 1 in, 3 out]
              n217 = Search 1D Array(1D array=w487, element=w485) -> (index of element=w482:i32)  [unwired: 1 out]
              n218 = Less Than 0?(x=w482) -> (x < 0?=w481:bool)
              n219 = And(x=w483, y=w481) -> (x .and. y?=w484:bool)
              n220 = case shown="True" w484 {
                tunnel: w487 -> [w491 w494]
                tunnel: [w491 w493] -> w486
                tunnel: w485 -> [_ w492]
                frame False {
                }
                frame True {
                  n221 = Build Array (concatenate)(w494, w492) -> (w493:string[])
                }
              }
            }
            n222 = for {
              tunnel: w473 -> [w479] mode=indexing
              n223 = call "Read_Traverse_Pos_File.vi"("Traverse Name"=w479) -> ("Tunnel Coordinates"=w478:dbl[])
              n224 = call "Read-Write_Check_Pos.vi"("Position input"=w478, "Mode"=enum16{"Read", "Write"}."Write", "Traverse Name"=w479) -> ()  [unwired: 1 out]
            }
          }
          frame Enabled {
          }
        }
      }
      frame "Experimental setup control" {
        n225 = global read "Trav_pos_global.vi" "Source Control?"() -> (w498:bool)
        n226 = Equal?(x=w501, y=User_Specific_mode."Run VI" ("Simulate/Run")) -> (x = y?=w500:bool)
        n227 = Or(x=w498, y=w500) -> (x .or. y?=w499:bool)
        n228 = case shown="True" w499 {
          tunnel: w498 -> [_ w505]
          frame False {
          }
          frame True {
            n229 = call "Exp_Setup_Control_remote.vi"("Dispersion?"=w505) -> ()  [unwired: 3 out]
          }
        }
        n230 = global write "Trav_pos_global.vi" "FFID Background"(T6 {"Start X"=nan, "Start Y"=nan, "Start Z"=nan, "End X"=nan, "End Y"=nan, "End Z"=nan, "No. of pts."=0, "Spacing"=enum."Linear", "Filename"=path "", "Tunnel Speed"=nan, "Averaging time (min)"=nan, "Extra Commands"="", "Specific Arguments"="", "Emission Rate (l/min)"=nan, "Trace Gas Concentration (%)"=nan, "Density Ratio"="", "Comments"="", "Row No"=0, "Row Type Selector"=enum."Blank Row", "Completion time"="", "Row Duration (mins)"=nan, "No. of Valid pts."=0, "Meas Setup File"=""} ("FFID Background")) -> ()
      }
      frame "Check source flowrates" {
        n231 = case shown="\"Run VI\"" w506 {
          tunnel: w507 -> [_ w516]
          frame "Check VI only", Default {
            n232 = Get Date/Time In Seconds() -> (seconds since 1Jan1904=w515:timestamp)
            n233 = global write "Trav_pos_global.vi" "Simulation Time"(w515) -> ()
          }
          frame "Run VI" {
            n234 = for {
              tunnel: w516 -> [w517] mode=indexing
              n235 = call "Set_Source.vi"("Source Status"=Client_Source_Status."Using", "Traverse line"=w517, "Simulate/Run"=User_Specific_mode."Check VI only") -> ()  [unwired: 1 in, 6 out]
            }
          }
        }
        n236 = Equal?(x=w506, y=User_Specific_mode."Run VI" ("Simulate/Run")) -> (x = y?=w510:bool)
        n237 = Increment(x=w512) -> (x+1=w508:T3)
        n238 = Select(t=w512, s=w510, f=w508) -> (s? t:f=w509:T3)
      }
      frame "Setup for running mode" {
        n239 = stacked-sequence {
          seq-local: [_ _ _ _ w553 _] -> [_ _ _ _ _ w571]
          tunnel: w523 -> [w528 _ _ w552 _ _]
          tunnel: w522 -> [_ _ w547 _ _ _]
          tunnel: [_ _ _ w550 _ _] -> w521
          tunnel: [_ _ _ _ w553 _] -> w520
          frame #0 {
            n240 = for {
              tunnel: w528 -> [w532] mode=indexing
              tunnel: [w529] -> w527 mode=indexing
              n241 = Unbundle By Name(w532) -> ("Row Type Selector"=w531:T8)
              n242 = Equal?(x=Multi_run_mode."Synchronize With:" ("Row Type Selector"), y=w531) -> (x = y?=w529:bool)
            }
            n243 = call "Setup_Environment.vi"() -> ()  [unwired: 1 in, 1 out]
            n244 = Or Array Elements(Boolean array=w527) -> (logical OR=w526:bool)
            n245 = case shown="True" w526 {
              frame False {
              }
              frame True {
                n246 = call "Declare_Sync_Client.vi"() -> ()  [unwired: 6 out]
              }
            }
          }
          frame #1 {
            n247 = Open VI Reference(vi path="Display_Trav_Views.vi" ("VI path")) -> (vi reference=w538:refnum<vi>, error out=w537:errorcluster)  [unwired: 1 in, 4 out]
            n248 = global write "Meas_global.vi" "Post Process"(Post_Process."Take New Data" ("Post Process")) -> ()
            n249 = property class="VI"(reference=w538, error in=w537, "Front Panel Window:Open"=FALSE) -> (reference out=w535:refnum<vi>, error out=w534:errorcluster)
            n250 = Close Reference(reference=w535, error in (no error)=w534) -> ()  [unwired: 1 out]
          }
          frame #2 {
            w542 = TRUE  # Start of Multi Run Prog
            w548 = TRUE
            n251 = Get Date/Time In Seconds() -> (seconds since 1Jan1904=w541:timestamp)
            n252 = To Double Precision Float(number=w541) -> (double precision float=w540:dbl)
            n253 = global write "Preference_global.vi" "Unblock Email"(w548) -> ()
            n254 = global write "Preference_global.vi" "Unblock SMS"(w548) -> ()
            n255 = global write "Meas_global.vi" "Start Time of experiment"(w540) -> ()
            n256 = local read "Command filename"() -> (w546:path)
            n257 = Path To String(path=w546) -> (string=w544:string)
            n258 = Concatenate Strings("Commencing a new multi run Prog having the setup filename of :" ("Message"), w544) -> (w543:string)
            n259 = call "Log_Current_row_to_Execute.vi"("Simulate/Run"=w547, "Message"=w543, "Start of Multi Run Prog"=w542) -> ()  [unwired: 2 in, 5 out]
          }
          frame #3 {
            n260 = call "Calc_Remaining_Time.vi"("Currently on Row"=-1, "Table In"=w552) -> ("Estimated Completion time"=w549:string, "Table Out"=w550:T6[])
            n261 = local write "Estimated Completion time"(w549) -> ()
            n262 = global write "Trav_pos_global.vi" "Estimated Completion time"(w549) -> ()
          }
          frame #4 {
            n263 = global read "Trav_pos_global.vi" "Source Control?"() -> (w554:bool)
            n264 = case shown="True" w554 {
              tunnel: [TRUE ("T button?") w559] -> w553
              frame False {
              }
              frame True {
                w560 = "EnFlo_Tunnel:Gas Solenoid:Status"
                n265 = Build Array(w560) -> (w563:string[])
                n266 = call "Get_Current_Scan_client.vi"("ADAM Ch Names"=w563) -> ("Numerical Values"=w562:dbl[])  [unwired: 3 out]
                n267 = Index Array(array=w562, index=0) -> (element=w558:dbl)
                n268 = Greater?(x=w558, y=0.5) -> (0:w556:bool)
                n269 = case shown="False" w556 {
                  tunnel: w560 -> [w569 _]
                  tunnel: [w564 TRUE ("T button?")] -> w559
                  frame False {
                    n270 = Format Into String(format string="The \"%s\" ADAM channel is showing that the blue gas button is not on.", w569) -> (resulting string=w567:string)  [unwired: 2 in, 1 out]
                    n271 = Two Button Dialog(message=w567, 1:"Stop" ("F button name (\"Cancel\")"), 2:"Continue" ("T button name (\"OK\")")) -> (T button?=w564:bool)
                  }
                  frame True {
                  }
                }
              }
            }
          }
          frame #5 {
            n272 = case shown="True" w571 {
              frame False {
              }
              frame True {
                n273 = call "Program_Active_Client.vi"("Mode"=enum16{"Program Active", "Traverse Level State"}."Traverse Level State", "Traverse level State"=Traverse_Level_State."Running") -> ()  [unwired: 1 in, 3 out]
              }
            }
          }
        }
      }
      frame "Skip Blank Rows" {
        n274 = stacked-sequence {
          tunnel: w578 -> [w581 w600]
          tunnel: w575 -> [w579 w596]
          frame #0 {
            n275 = Decrement(x=w581) -> (x-1=w580:i32)
            n276 = while {
              tunnel: w579 -> [w591]
              tunnel: w580 -> [w585]
              stop <- w582 continue-if-true
              n277 = local read "Currently on Row"() -> (w587:i32)
              n278 = Increment(x=w587) -> (x+1=w586:i32)
              n279 = Less?(x=w586, y=w585) -> (x < y?=w584:bool)
              n280 = Index Array(array=w591, index=w586) -> (element=w590:T6)
              n281 = Unbundle By Name(w590) -> ("Row Type Selector"=w589:T8)
              n282 = Equal?(x=Multi_run_mode."Blank Row" ("Row Type Selector"), y=w589) -> (x = y?=w583:bool)
              n283 = case shown="True" w583 {
                tunnel: w586 -> [_ w592]
                frame False {
                }
                frame True {
                  n284 = local write "Currently on Row"(w592) -> ()
                }
              }
              n285 = And(x=w583, y=w584) -> (x .and. y?=w582:bool)
            }
          }
          frame #1 {
            n286 = local read "Currently on Row"() -> (w598:i32)
            n287 = Increment(x=w598) -> (x+1=w597:i32)
            n288 = Index Array(array=w596, index=w597) -> (element=w599:T6)
            n289 = Unbundle By Name(w599) -> ("Row Type Selector"=w595:T8)
            n290 = Equal?(x=Multi_run_mode."Turn Off Row Repeating" ("Row Type Selector"), y=w595) -> (x = y?=w593:bool)
            n291 = while {
              shift-right: [w609] -> _
              shift-left: _ -> [w608]
              tunnel: w600 -> [w605]
              tunnel: w598 -> [w609]
              tunnel: w593 -> [w602]
              stop <- TRUE stop-if-true
              n292 = Decrement(x=w605) -> (x-1=w610:i32)
              n293 = Equal?(x=w609, y=w610) -> (x = y?=w603:bool)
              n294 = Not Equal?(x=w609, y=w608) -> (x != y?=w607:bool)
              n295 = Or(x=w602, y=w603) -> (x .or. y?=w601:bool)
              n296 = And(x=w607, y=w601) -> (x .and. y?=w606:bool)
              n297 = case shown="True" w606 {
                tunnel: w605 -> [_ w611]
                frame False {
                }
                frame True {
                  n298 = Initialize Array(timestamp(0 s since 1904-01-01) ("seconds since 1Jan1904"), w611) -> (w613:timestamp[])
                  n299 = global write "Trav_pos_global.vi" "Row completion times"(w613) -> ()
                }
              }
            }
          }
        }
      }
      frame "Which row to execute next" {
        # "Rep?"
        # "Repeat\nRow"
        n300 = local read "Currently on Row"() -> (w614:i32)
        n301 = stacked-sequence {
          seq-local: [_ w653 _] -> [_ _ w689]
          seq-local: [_ w652 _] -> [_ _ w690]
          seq-local: [w623 _ _] -> [_ w651 _]
          seq-local: [_ w648 _] -> [_ _ w683]
          tunnel: [w628 _ _] -> w620
          tunnel: w619 -> [w628 w655 w697]
          tunnel: w618 -> [_ _ w695]
          tunnel: w617 -> [_ w650 w696]
          tunnel: [_ _ w692] -> w616
          tunnel: w615 -> [_ _ w691]
          tunnel: w614 -> [w625 w647 w682]
          frame #0 {
            n302 = Array Size(array=w628) -> (size(s)=w627:i32)
            n303 = Decrement(x=w627) -> (x-1=w626:i32)
            n304 = Increment(x=w625) -> (x+1=w624:i32)
            n305 = while {
              tunnel: w624 -> [w632]
              tunnel: w628 -> [w644] mode=indexing
              tunnel: Multi_run_mode."Turn Off Row Repeating" ("Row Type Selector") -> [w643]
              tunnel: w626 -> [w639]
              tunnel: [w634] -> w623
              i -> [w636]
              stop <- w642 continue-if-true
              n306 = Less?(x=w636, y=w632) -> (x < y?=w637:bool)
              n307 = Unbundle By Name(w644) -> ("Row Type Selector"=w641:T8)
              n308 = Less?(x=w636, y=w639) -> (x < y?=w638:bool)
              n309 = Equal?(x=w636, y=w632) -> (x = y?=w633:bool)
              n310 = Equal?(x=w643, y=w641) -> (x = y?=w635:bool)
              n311 = case shown="True" w635 {
                tunnel: [TRUE w646] -> w634
                tunnel: w633 -> [_ w646]
                frame False {
                }
                frame True {
                }
              }
              n312 = Not(x=w635) -> (.not. x?=w640:bool)
              n313 = Compound Arithmetic op=AND(w640, w637, w638) -> (w642:bool)
            }
            n314 = global write "Trav_pos_global.vi" "Currently on point"(0 ("Currently on point")) -> ()
            n315 = global write "Trav_pos_global.vi" "Paused During Row?"(FALSE ("Paused During Row?")) -> ()
            n316 = global write "Trav_pos_global.vi" "Repeat Rows?"(w623) -> ()
          }
          frame #1 {
            n317 = global read "Trav_pos_global.vi" "Row completion times"() -> (w654:timestamp[])
            n318 = global read "Extra_Commands_Global.vi" "Minutes Before Repeating Row"() -> (w649:string)
            n319 = case shown="\"Run VI\"" w650 {
              tunnel: [w656 w657] -> w648
              frame "Check VI only" {
                n320 = global read "Trav_pos_global.vi" "Simulation Time"() -> (w656:timestamp)
              }
              frame "Run VI" {
                n321 = Get Date/Time In Seconds() -> (seconds since 1Jan1904=w657:timestamp)
                n322 = global write "Trav_pos_global.vi" "Simulation Time"(w657) -> ()
              }
            }
            n323 = while {
              tunnel: w655 -> [w667] mode=indexing
              tunnel: w654 -> [w670]
              tunnel: w648 -> [w669]
              tunnel: [w660] -> w653
              tunnel: [w659] -> w652
              tunnel: w651 -> [w663]
              tunnel: w647 -> [w661]
              tunnel: w649 -> [w658]
              i -> [w659]
              stop <- w666 continue-if-true
              n324 = Unbundle By Name(w667) -> ("Extra Commands"=w671:string)
              n325 = call "Extra_Commands.vi"("String to Search"=w671, "Command"=w658) -> ("Numeric Value"=w668:dbl, "Command Found"=w664:bool)  [unwired: 1 in, 3 out]
              n326 = And(x=w663, y=w664) -> (x .and. y?=w662:bool)
              n327 = case shown="True" w662 {
                tunnel: w670 -> [_ w677]
                tunnel: w669 -> [_ w678]
                tunnel: w659 -> [_ w676]
                tunnel: w668 -> [_ w674]
                tunnel: [FALSE w673] -> w660
                frame False {
                }
                frame True {
                  n328 = Index Array(array=w677, index=w676) -> (element=w679:timestamp)
                  n329 = Subtract(x=w678, y=w679) -> (x-y=w680:dbl)
                  n330 = Divide(x=w680, y=60.0) -> (x/y=w675:dbl)
                  n331 = Greater?(x=w675, y=w674) -> (0:w673:bool)
                }
              }
              n332 = Less?(x=w659, y=w661) -> (x < y?=w665:bool)
              n333 = Compound Arithmetic op=AND(invert w660, w665) -> (w666:bool)
            }
          }
          frame #2 {
            n334 = Not Equal?(x=w682, y=w690) -> (x != y?=w688:bool)
            n335 = And(x=w689, y=w688) -> (x .and. y?=w687:bool)
            n336 = case shown="False" w687 {
              tunnel: w690 -> [_ w723]
              tunnel: w682 -> [w719 w725]
              tunnel: [w718 w724] -> w693
              tunnel: [w718 w723] -> w684
              tunnel: w695 -> [w721 _]
              tunnel: [w717 TRUE] -> w694
              frame False {
                n337 = Increment(x=w719) -> (x+1=w720:i32)
                n338 = Greater?(x=w721, y=w720) -> (0:w717:bool)
                n339 = Select(t=w720, s=w717, f=w719) -> (s? t:f=w718:i32)
              }
              frame True {
                n340 = Greater?(x=w725, y=w723) -> (0:w726:bool)
                n341 = Select(t=w725, s=w726, f=w723) -> (s? t:f=w724:i32)
              }
            }
            n342 = global read "Trav_pos_global.vi" "Row completion times"() -> (w686:timestamp[])
            n343 = case shown="True" w694 {
              tunnel: w684 -> [_ w705]
              tunnel: w697 -> [_ w711]
              tunnel: w696 -> [w699 w703]
              tunnel: w693 -> [_ w709]
              tunnel: [w698 w708] -> w692
              tunnel: w691 -> [_ w708]
              frame False {
                n344 = case shown="\"Run VI\"" w699 {
                  tunnel: [Multi_Run_Case."Show jumped positions" ("Multi Run Case") Multi_Run_Case."Shut down source etc" ("Multi Run Case")] -> w698
                  frame "Check VI only" {
                  }
                  frame "Run VI" {
                  }
                }
              }
              frame True {
                n345 = Index Array(array=w711, index=w705) -> (element=w707:T6)
                n346 = Bundle By Name(cluster=w707, "Row No"=w705) -> (w706:T6)
                n347 = global write "Trav_pos_global.vi" "Meas Setup Number"(0 ("Meas Setup Number")) -> ()
                n348 = Build Array(w709) -> (w710:i32[])
                n349 = case shown="\"Run VI\"" w703 {
                  tunnel: w703 -> [_ w715]
                  tunnel: w706 -> [w712 w714]
                  tunnel: [w712 w713] -> w702
                  frame "Check VI only" {
                  }
                  frame "Run VI" {
                    n350 = call "Log_Current_row_to_Execute.vi"("Simulate/Run"=w715, "Start of Multi Run Prog"=FALSE, "Traverse line in"=w714) -> ("Traverse line Out"=w713:T6)  [unwired: 2 in, 4 out]
                  }
                }
                n351 = property on="Table" class="Arr (strict)"("Index Values"=w710) -> ()  [unwired: 2 in, 2 out]
                n352 = global write "Trav_pos_global.vi" "Current Row"(w702) -> ()
                "Currently on Row" <- w709
              }
            }
            n353 = Replace Array Subset(array=w686, new element=w683, index=w684) -> (w685:timestamp[])
            n354 = global write "Trav_pos_global.vi" "Row completion times"(w685) -> ()
          }
        }
      }
      frame "Evaluate IF Statement" {
        n355 = global read "Trav_pos_global.vi" "Current Row"() -> (w731:T6)
        n356 = Unbundle By Name(w731) -> ("Extra Commands"=w734:string)
        n357 = global read "Extra_Commands_Global.vi" "If Command"() -> (w737:string)
        n358 = call "Extra_Commands.vi"("String to Search"=w734, "Command"=w737) -> ("String Value"=w736:string, "Command Found"=w728:bool)  [unwired: 1 in, 3 out]
        n359 = Equal?(x=w732, y=User_Specific_mode."Run VI" ("Simulate/Run")) -> (x = y?=w727:bool)
        n360 = And(x=w728, y=w727) -> (x .and. y?=w729:bool)
        n361 = case shown="True" w729 {
          tunnel: w736 -> [_ w747]
          tunnel: [w743 w746] -> w730
          frame False {
            w743 = TRUE  # Execute Row?
          }
          frame True {
            n362 = call "Get_array_values_fr_String.vi"("String Value"=w747) -> ("Numeric Array"=w745:dbl[], "String array"=w744:string[])
            n363 = Index Array(array=w744, index=0 ("Index")) -> (element=w748:string)
            n364 = case shown="\"Global Value Between\"" w748 {
              tunnel: w747 -> [w753 _ _ _]
              tunnel: [w752 w754 w764 TRUE ("Execute Row?")] -> w746
              tunnel: w745 -> [_ w760 w778 _]
              tunnel: w744 -> [_ _ w772 _]
              frame "Time Between" {
                n365 = Get Date/Time In Seconds() -> (seconds since 1Jan1904=w750:timestamp)
                n366 = To Double Precision Float(number=w750) -> (double precision float=w751:dbl)
                n367 = call "If_Time_arguments.vi"("seconds since 1Jan1904"=w751, "String Value"=w753) -> ("Execute Row?"=w752:bool)  [unwired: 2 out]
              }
              frame "Global Value Between" {
                n368 = global read "Extra_Commands_Global.vi" "If command global value"() -> (w755:dbl)
                n369 = Index Array(array=w760, index=1 ("Index")) -> (element=w758:dbl)
                n370 = Index Array(array=w760, index=2 ("Index")) -> (element=w759:dbl)
                n371 = Max & Min(x=w758, y=w759) -> (max(x,y)=w757:dbl, min(x,y)=w756:dbl)
                n372 = In Range and Coerce(upper limit=w757, x=w755, lower limit=w756) -> (In Range?=w754:bool)  [unwired: 1 out]
              }
              frame "ADAM Channel Between" {
                n373 = Index Array(array=w772, index=1 ("Index")) -> (element=w771:string)
                n374 = Build Array(w771) -> (w770:string[])
                n375 = Index Array(array=w778, index=2 ("Index")) -> (element=w776:dbl)
                n376 = Index Array(array=w778, index=3 ("Index")) -> (element=w777:dbl)
                n377 = Max & Min(x=w776, y=w777) -> (max(x,y)=w775:dbl, min(x,y)=w774:dbl)
                n378 = call "Get_Current_Scan_client.vi"("ADAM Ch Names"=w770) -> ("Numerical Values"=w768:dbl[])  [unwired: 3 out]
                n379 = Index Array(array=w768, index=0 ("Index")) -> (element=w767:dbl)
                n380 = In Range and Coerce(upper limit=w775, x=w767, lower limit=w774) -> (In Range?=w765:bool)  [unwired: 1 out]
                n381 = Not A Number/Path/Refnum?(number/path/refnum=w767) -> (NaN/Path/Refnum?=w766:bool)
                n382 = Select(t=TRUE, s=w766, f=w765) -> (s? t:f=w764:bool)
              }
              frame "No Match", Default {
              }
            }
          }
        }
        n383 = Select(t=w740, s=w730, f=Multi_Run_Case."Calculate Row TIme" ("Multi Run Case")) -> (s? t:f=w739:T3)
      }
      frame "Perform Measurement Setup" {
        n384 = global read "Trav_pos_global.vi" "Current Row"() -> (w784:T6)
        n385 = case shown="\"Run VI\"" w783 {
          tunnel: w784 -> [_ w789]
          tunnel: w783 -> [_ w788]
          frame "Check VI only" {
          }
          frame "Run VI" {
            n386 = stacked-sequence {
              tunnel: w789 -> [w792 _]
              tunnel: w788 -> [w790 _]
              frame #0 {
                n387 = Unbundle By Name(w792) -> ("Extra Commands"=w791:string)
                n388 = call "Pause_for_server_ch_val.vi"("Extra command string"=w791, "Simulate/Run"=w790) -> ()  [unwired: 2 out]
              }
              frame #1 {
                n389 = Get Date/Time In Seconds() -> (seconds since 1Jan1904=w793:timestamp)
                n390 = To Double Precision Float(number=w793) -> (double precision float=w794:dbl)
                n391 = global write "Trav_pos_global.vi" "Start of Row time (Sec)"(w794) -> ()
              }
            }
          }
        }
      }
      frame "Set Measurement Conditions" {
        w800 = TRUE  # Row Completed
        w799 = FALSE  # Row Completed
        n392 = global read "Trav_pos_global.vi" "Current Row"() -> (w797:T6)
        n393 = Unbundle By Name(w797) -> ("Row Type Selector"=w802:T8)
        n394 = case shown="\"Run VI Named:\"" w802 {
          tunnel: [TRUE FALSE TRUE TRUE TRUE TRUE FALSE TRUE FALSE w851 FALSE FALSE FALSE] -> w807
          tunnel: w797 -> [w815 w818 w821 w824 w827 w830 w833 w836 w845 w850 w873 w876 w879]
          tunnel: [w815 w818 w821 w824 w827 w830 w833 w836 w844 w849 w873 w876 w879] -> w803
          tunnel: [w814 w817 w820 w823 w826 w829 w832 w835 w840 w847 w872 w875 w878] -> w801
          tunnel: w800 -> [w814 _ w820 w823 w826 _ _ _ _ w847 w872 w875 w878]
          tunnel: w799 -> [_ w817 _ _ _ w829 w832 w835 w840 _ _ _ _]
          tunnel: w796 -> [_ _ _ _ _ _ _ _ _ w848 _ _ _]
          frame "Move Traverse Only" {
          }
          frame "Check Beam Power" {
          }
          frame "Set Tunnel Speed Only" {
          }
          frame "Set Source Only" {
          }
          frame "Set Measurement Conditions" {
          }
          frame "Single Measurement" {
          }
          frame "Vertical Profile", Default {
          }
          frame "Scanning Valve Measurement" {
          }
          frame "Run VI Named:" {
            n395 = global read "Extra_Commands_Global.vi" "Skip Source Demand"() -> (w843:string)
            n396 = global read "Extra_Commands_Global.vi" "Establish Exp Conditions (s)"() -> (w839:string)
            n397 = Unbundle By Name(w845) -> ("Extra Commands"=w842:string)
            n398 = Concatenate Strings(w839, " = 0" ("Substring"), w843, w842) -> (w841:string)
            n399 = Bundle By Name(cluster=w845, "Extra Commands"=w841) -> (w844:T6)
          }
          frame "Send Message" {
            n400 = stacked-sequence {
              seq-local: [w852 _ _ _] -> [_ w857 _ _]
              tunnel: [_ _ _ FALSE] -> w851
              tunnel: w850 -> [_ w860 w866 w869]
              tunnel: [_ _ _ w869] -> w849
              tunnel: w848 -> [w853 _ _ _]
              frame #0 {
                n401 = Equal?(x=User_Specific_mode."Run VI" ("Simulate/Run"), y=w853) -> (x = y?=w852:bool)
              }
              frame #1 {
                n402 = Unbundle By Name(w860) -> ("Specific Arguments"=w858:string, "Filename"=w856:path)
                n403 = Build Array(w856) -> (w855:path[])
                n404 = case shown="True" w857 {
                  tunnel: "Message" ("Error Type") -> [_ w863]
                  tunnel: w858 -> [_ w862]
                  tunnel: w855 -> [_ w861]
                  frame False {
                  }
                  frame True {
                    n405 = call "Email_Text_Files.vi"("Filenames"=w861, "message"=w862, "subject ([No Subject])"=w863) -> ()
                  }
                }
              }
              frame #2 {
                n406 = global read "Extra_Commands_Global.vi" "Establish Exp Conditions (s)"() -> (w868:string)
                n407 = Unbundle By Name(w866) -> ("Extra Commands"=w867:string)
                n408 = call "Extra_Commands.vi"("String to Search"=w867, "Command"=w868) -> ("Numeric Value"=w864:dbl)  [unwired: 1 in, 4 out]
                n409 = call "Wait_Seconds_with_display.vi"("Message"="In Send Message Row", "Seconds to wait"=w864) -> ()  [unwired: 2 out]
              }
              frame #3 {
              }
            }
          }
          frame "Fall Back to this Row" {
          }
          frame "Turn Off Row Repeating" {
          }
          frame "Blank Row" {
          }
        }
        n410 = case shown="True" w807 {
          tunnel: w803 -> [_ w881]
          tunnel: w796 -> [_ w885]
          tunnel: [Multi_Run_Status."Continue" ("Status") w882] -> w795
          frame False {
          }
          frame True {
            w884 = 1  # Currently on Point
            n411 = call "Program_Active.vi"() -> ()  [unwired: 1 in]
            n412 = call "Set_Measurement_Conditions.vi"("Simulate/Run"=w885, "Currently on Point"=w884, "Traverse line"=w881) -> ("Status Cluster"=w883:T22)  [unwired: 2 out]
            n413 = Unbundle By Name(w883) -> ("Status"=w882:T2)
          }
        }
        n414 = case shown="\"Continue\"" w795 {
          tunnel: [w811 Multi_Run_Case."Calculate Row TIme" ("Multi Run Case")] -> w806
          tunnel: w805 -> [w812 _]
          tunnel: w801 -> [w809 _]
          frame "Continue" {
            n415 = Select(t=Multi_Run_Case."Calculate Row TIme" ("Multi Run Case"), s=w809, f=w812) -> (s? t:f=w811:T3)
          }
          frame "Jump to Next Point", Default {
          }
        }
        n416 = local write "Status"(w795) -> ()
      }
      frame "Execute Row" {
        n417 = global read "Trav_pos_global.vi" "Current Row"() -> (w887:T6)
        n418 = stacked-sequence {
          tunnel: w888 -> [w892 w903 w905]
          tunnel: w887 -> [w893 w900 w904]
          frame #0 {
            n419 = case shown="\"Check VI only\"" w892 {
              tunnel: w893 -> [w896 _]
              tunnel: w892 -> [w895 _]
              frame "Check VI only" {
                n420 = Unbundle By Name(w896) -> ("Extra Commands"=w897:string, "Row No"=w899:i32, "Meas Setup File"=w894:string)
                n421 = call "Skip_If Sd_Error_Below.vi"("String to Search"=w897, "Simulate/Run"=w895, "Measurement setup Applied?"=TRUE, "Row Number"=w899, "Measurement Setup File"=w894) -> ()  [unwired: 5 out]
              }
              frame "Run VI" {
              }
            }
          }
          frame #1 {
            n422 = call "Execute_Row.vi"("Simulate/Run"=w903, "Traverse line"=w900) -> ("Status"=w902:T2, "Traverse line out"=w901:T6)  [unwired: 2 out]
            n423 = global write "Trav_pos_global.vi" "Current Row"(w901) -> ()
            n424 = local write "Status"(w902) -> ()
          }
          frame #2 {
            w908 = FALSE  # Empty list
            n425 = call "Remember_RD_Folders.vi"("Empty list"=w908) -> ("List of Folders"=w907:path[])  [unwired: 1 in]
            n426 = for {
              tunnel: w904 -> [w913]
              tunnel: w907 -> [w912] mode=indexing
              tunnel: "Muti_Run_Log.xls" ("name or relative path") -> [w910]
              tunnel: w905 -> [w909]
              n427 = Build Path(base path=w912, name or relative path=w910) -> (appended path=w911:path)
              n428 = call "Log_Current_row_to_Execute.vi"("Simulate/Run"=w909, "Start of Multi Run Prog"=FALSE, "Traverse line in"=w913, "Multi Run Log File"=w911) -> ()  [unwired: 1 in, 5 out]
            }
          }
        }
      }
      frame "Calculate Row TIme" {
        n429 = global read "Trav_pos_global.vi" "Paused During Row?"() -> (w918:bool)
        n430 = local read "Status"() -> (w921:T2)
        n431 = global read "Trav_pos_global.vi" "Current Row"() -> (w917:T6)
        n432 = Equal?(x=w921, y=Multi_Run_Status."Continue" ("Status")) -> (x = y?=w920:bool)
        n433 = Equal?(x=w923, y=User_Specific_mode."Run VI" ("Simulate/Run")) -> (x = y?=w919:bool)
        n434 = Compound Arithmetic op=AND(w920, w919, invert w918) -> (w916:bool)
        n435 = case shown="False" w916 {
          tunnel: w917 -> [w936 w947]
          frame False {
            n436 = global read "Trav_pos_global.vi" "Simulation Time"() -> (w937:timestamp)
            n437 = To Double Precision Float(number=w937) -> (double precision float=w931:dbl)
            n438 = call "Calculate_Row_Time.vi"("Row Start Time (Sec Since 1904)"=w931, "Multi Run Row"=w936) -> ("Scalable Time (Sec)"=w934:dbl, "Fixed Time (Sec)"=w932:dbl)
            n439 = call "Overhead_Factor.vi"("Mode"=Overhead."Read Current Overhead") -> ("Current Overhead Factor"=w935:dbl)  [unwired: 3 in]
            n440 = Multiply(x=w935, y=w934) -> (x*y=w933:dbl)
            n441 = Add(x=w932, y=w933) -> (x+y=w928:dbl)
            n442 = global write "Trav_pos_global.vi" "Start of Row time (Sec)"(w928) -> ()
            n443 = Add(x=w931, y=w928) -> (x+y=w930:dbl)
            n444 = To Time Stamp(1:w930) -> (0:w929:timestamp)
            n445 = global write "Trav_pos_global.vi" "Simulation Time"(w929) -> ()
          }
          frame True {
            n446 = global read "Trav_pos_global.vi" "Start of Row time (Sec)"() -> (w945:dbl)
            n447 = Get Date/Time In Seconds() -> (seconds since 1Jan1904=w940:timestamp)
            n448 = To Double Precision Float(number=w940) -> (double precision float=w939:dbl)
            n449 = call "Calculate_Row_Time.vi"("Row Start Time (Sec Since 1904)"=w945, "Multi Run Row"=w947) -> ("Scalable Time (Sec)"=w941:dbl, "Fixed Time (Sec)"=w943:dbl)
            n450 = Subtract(x=w939, y=w945) -> (x-y=w944:dbl)
            n451 = Subtract(x=w944, y=w943) -> (x-y=w942:dbl)
            n452 = call "Overhead_Factor.vi"("Sum of Ideal times (Sec)"=w941, "Sum of Actual times (Sec)"=w942, "Mode"=Overhead."Update total times") -> ()  [unwired: 1 in, 1 out]
          }
        }
      }
      frame "Update time estimate" {
        n453 = global read "Trav_pos_global.vi" "Current Row"() -> (w951:T6)
        n454 = Unbundle By Name(w951) -> ("Row No"=w949:i32)
        n455 = local read "Currently on Row"() -> (w950:i32)
        n456 = Equal?(x=w949, y=w950) -> (x = y?=w948:bool)
        n457 = case shown="\"Run VI\"" w954 {
          tunnel: w957 -> [w965 w986]
          tunnel: [w964 w982] -> w956
          tunnel: w953 -> [_ w988]
          tunnel: [w963 w987] -> w952
          tunnel: w950 -> [w961 w981]
          tunnel: w951 -> [w962 w985]
          tunnel: w948 -> [w960 w984]
          frame "Check VI only" {
            n458 = global read "Trav_pos_global.vi" "Simulation Time"() -> (w967:timestamp)
            n459 = To Double Precision Float(number=w967) -> (double precision float=w966:dbl)
            n460 = call "Sec_to_date_filename.vi"("seconds"=w966) -> ("Day"=w969:string, "Time"=w968:string)  [unwired: 2 out]
            n461 = Concatenate Strings(w968, "  " ("Substring"), w969) -> (w963:string)
            n462 = case shown="True" w960 {
              tunnel: w961 -> [_ w980]
              tunnel: w965 -> [w971 w979]
              tunnel: [w971 w977] -> w964
              tunnel: w963 -> [_ w976]
              tunnel: w962 -> [_ w975]
              frame False {
              }
              frame True {
                n463 = global read "Trav_pos_global.vi" "Start of Row time (Sec)"() -> (w974:dbl)
                n464 = Divide(x=w974, y=60.0) -> (x/y=w972:dbl)
                n465 = Bundle By Name(cluster=w975, "Completion time"=w976, "Row Duration (mins)"=w972) -> (w978:T6)
                n466 = Replace Array Subset(array=w979, new element=w978, index=w980) -> (w977:T6[])
              }
            }
          }
          frame "Run VI" {
            n467 = case shown="True" w984 {
              tunnel: w981 -> [_ w995]
              tunnel: w986 -> [w991 w994]
              tunnel: w985 -> [_ w993]
              tunnel: [w991 w992] -> w983
              frame False {
              }
              frame True {
                n468 = Replace Array Subset(array=w994, new element=w993, index=w995) -> (w992:T6[])
              }
            }
            n469 = call "Calc_Remaining_Time.vi"("Currently on Row"=w981, "Table In"=w983) -> ("Table Out"=w982:T6[])  [unwired: 1 out]
            n470 = Decrement(x=w988) -> (x-1=w990:i32)
            n471 = Index Array(array=w982, index=w990) -> (element=w989:T6)
            n472 = Unbundle By Name(w989) -> ("Completion time"=w987:string)
          }
        }
        "Estimated Completion time" <- w952
        n473 = global write "Trav_pos_global.vi" "Estimated Completion time"(w952) -> ()
      }
      frame "Pause Multi Run Program" {
        n474 = while {
          tunnel: "Pause" -> [w1007]
          tunnel: [w1010] -> w1002
          tunnel: w1001 -> [w1009]
          tunnel: w999 -> [w1008]
          shift-right: [w1007] -> _
          shift-left: _ -> [w1006]
          stop <- TRUE stop-if-true
          n475 = case shown="True" w1007 {
            tunnel: [w1011 w1016] -> w1010
            tunnel: w1009 -> [w1011 w1014]
            tunnel: w1008 -> [_ w1015]
            tunnel: w1007 -> [_ w1013]
            tunnel: w1006 -> [_ w1012]
            frame False {
            }
            frame True {
              n476 = stacked-sequence {
                tunnel: w1014 -> [_ _ _ _ w1031]
                tunnel: [_ _ _ _ w1032] -> w1016
                tunnel: w1015 -> [w1018 _ _ _ _]
                tunnel: w1013 -> [_ _ _ w1027 _]
                tunnel: w1012 -> [_ _ _ w1026 _]
                frame #0 {
                  n477 = Quotient & Remainder(x=w1018, y=15) -> (x-y*floor(x/y)=w1017:i32)  [unwired: 1 out]
                  n478 = case shown="0" w1017 {
                    frame 0 {
                      n479 = Current VI's Path() -> (path=w1020:path)
                      n480 = call "Bring_to_front.vi"("path"=w1020) -> ()
                    }
                    frame 1, Default {
                    }
                  }
                }
                frame #1 {
                  n481 = global write "Trav_pos_global.vi" "Paused During Row?"(TRUE ("Paused During Row?")) -> ()
                  "Pause message" <- "Multi Run Program Paused!!!!" ("Pause message")
                }
                frame #2 {
                  n482 = property on="Pause message" class="Str"("Visible"=TRUE) -> ()  [unwired: 2 in, 2 out]
                  n483 = Wait Until Next ms Multiple(millisecond multiple=u32 1500) -> ()  [unwired: 1 out]
                }
                frame #3 {
                  n484 = Compound Arithmetic op=AND(w1027, invert w1026) -> (w1025:bool)
                  n485 = case shown="True" w1025 {
                    frame False {
                    }
                    frame True {
                      n486 = call "Program_Active_Client.vi"("Mode"=enum16{"Program Active", "Traverse Level State"}."Program Active", "Time till next contact (Sec)"=12000.0, "Traverse level State"=Traverse_Level_State."Running") -> ()  [unwired: 3 out]
                    }
                  }
                }
                frame #4 {
                  n487 = property on="Pause message" class="Str"("Visible"=FALSE) -> ()  [unwired: 2 in, 2 out]
                  n488 = Wait Until Next ms Multiple(millisecond multiple=u32 1500) -> ()  [unwired: 1 out]
                  n489 = Decrement(x=w1031) -> (x-1=w1032:T3)
                }
              }
            }
          }
        }
        n490 = call "Overhead_Factor.vi"("Mode"=Overhead."Read Current Overhead") -> ("Current Overhead Factor"=→"Current Overhead Factor":dbl)  [unwired: 3 in]
      }
      frame "Do Another Row?" {
        w1045 = Multi_Run_Status."Terminate Run" ("Status")
        n491 = case shown="False" "Stop after Repeats" {
          tunnel: [w1053 w1054] -> w1039
          tunnel: w1035 -> [_ w1055]
          frame False {
            n492 = local read "Currently on Row"() -> (w1053:i32)
            n493 = Increment(x=w1053) -> (x+1=→"Last Row Run":i32)
          }
          frame True {
            n494 = Decrement(x=w1055) -> (x-1=w1054:i32)
            n495 = local write "Currently on Row"(w1054) -> ()
          }
        }
        n496 = case shown="False" "stop" {
          tunnel: [w1056 w1057] -> w1046
          tunnel: w1045 -> [_ w1057]
          frame False {
            n497 = local read "Status"() -> (w1056:T2)
          }
          frame True {
            n498 = local write "Status"(w1057) -> ()
          }
        }
        n499 = Not Equal?(x=w1046, y=w1045) -> (x != y?=w1044:bool)
        n500 = Increment(x=w1039) -> (x+1=w1038:i32)
        n501 = Index Array(array=w1040, index=w1038) -> (element=w1037:T6)
        n502 = Unbundle By Name(w1037) -> ("Row Type Selector"=w1043:T8)
        n503 = Equal?(x=w1043, y=Multi_run_mode."Turn Off Row Repeating" ("Row Type Selector")) -> (x = y?=w1041:bool)
        n504 = case shown="True" w1044 {
          tunnel: [w1058 w1062] -> w1050
          tunnel: w1039 -> [_ _]
          tunnel: w1049 -> [w1059 _]
          tunnel: w1040 -> [_ _]
          tunnel: w1046 -> [_ w1063]
          tunnel: w1035 -> [_ _]
          tunnel: w1041 -> [_ _]
          frame False {
            n505 = case shown="\"Check VI only\"" w1059 {
              tunnel: [Multi_Run_Case."Show jumped positions" ("Multi Run Case") Multi_Run_Case."Shut down source etc" ("Multi Run Case")] -> w1058
              frame "Check VI only" {
              }
              frame "Run VI" {
              }
            }
          }
          frame True {
            n506 = case shown="\"Jump To Fall Back\"" w1063 {
              tunnel: [Multi_Run_Case."Skip Blank Rows" ("Multi Run Case") Multi_Run_Case."Find Next Fall Back Row" ("Multi Run Case")] -> w1062
              frame "Continue", Default {
              }
              frame "Jump To Fall Back" {
              }
            }
          }
        }
      }
      frame "Find Next Fall Back Row" {
        n507 = local read "Currently on Row"() -> (w1067:i32)
        n508 = Increment(x=w1067) -> (x+1=w1066:i32)
        n509 = Index Array(array=w1075, index=w1067) -> (element=w1076:T6)
        n510 = Array Size(array=w1075) -> (size(s)=w1074:i32)
        n511 = Unbundle By Name(w1076) -> ("Row Type Selector"=w1070:T8)
        n512 = Greater?(x=w1074, y=w1066) -> (0:w1073:bool)
        n513 = Equal?(x=w1070, y=Multi_run_mode."Fall Back to this Row" ("Mode")) -> (x = y?=w1068:bool)
        n514 = case shown="True" w1073 {
          tunnel: [Multi_Run_Case."Skip Blank Rows" ("Multi Run Case") w1083] -> w1072
          tunnel: w1068 -> [_ w1079]
          tunnel: w1067 -> [_ w1080]
          frame False {
          }
          frame True {
            n515 = case shown="False" w1079 {
              tunnel: w1080 -> [w1085 _]
              frame False {
                n516 = Increment(x=w1085) -> (x+1=w1084:i32)
                n517 = local write "Currently on Row"(w1084) -> ()
              }
              frame True {
              }
            }
            n518 = Select(t=Multi_Run_Case."Skip Blank Rows" ("Multi Run Case"), s=w1079, f=Multi_Run_Case."Find Next Fall Back Row" ("Multi Run Case")) -> (s? t:f=w1083:T3)
          }
        }
      }
      frame "Shut down source etc" {
        n519 = for {
          tunnel: w1105 -> [w1124] mode=indexing
          tunnel: Multi_run_mode."Synchronize With:" ("Mode") -> [w1122]
          tunnel: [w1121] -> w1107 mode=indexing
          n520 = Unbundle By Name(w1124) -> ("Row Type Selector"=w1123:T8)
          n521 = Equal?(x=w1123, y=w1122) -> (x = y?=w1121:bool)
        }
        n522 = call "Overhead_Factor.vi"("Mode"=Overhead."Re Scale totals to 3 hrs") -> ()  [unwired: 3 in, 1 out]
        n523 = local read "Status"() -> (w1093:T2)
        n524 = call "Set_Source.vi"("Source Status"=Client_Source_Status."Not Using", "Simulate/Run"=w1096) -> ("Status Cluster"=w1097:T22)  [unwired: 2 in, 5 out]
        n525 = call "Program_Active_Client.vi"("Mode"=enum16{"Program Active", "Traverse Level State"}."Traverse Level State", "Traverse level State"=Traverse_Level_State."Complete") -> ()  [unwired: 1 in, 3 out]
        n526 = global read "Meas_global.vi" "Start Time of experiment"() -> (w1103:dbl)
        n527 = Equal?(x=w1093, y=Multi_Run_Status."Terminate Run" ("Status")) -> (x = y?=w1091:bool)
        n528 = call "Prog_Status_Handler.vi"("Status Cluster"=w1097, "Simulate/Run"=w1096) -> ()  [unwired: 2 out]
        n529 = global read "Meas_global.vi" "LDA data"() -> (w1112:enum16{"No LDA data", "Take LDA data"})
        n530 = Or Array Elements(Boolean array=w1107) -> (logical OR=w1094:bool)
        n531 = Get Date/Time In Seconds() -> (seconds since 1Jan1904=w1086:timestamp)
        n532 = Compound Arithmetic op=AND(w1094, invert w1091) -> (w1095:bool)
        n533 = To Double Precision Float(number=w1086) -> (double precision float=w1104:dbl)
        n534 = case shown="\"Take LDA data\"" w1112 {
          frame "No LDA data" {
          }
          frame "Take LDA data" {
            w1125 = FALSE  # High Voltage
            w1130 = 0.0  # Input
            n535 = global read "LDA_meas_global_2.vi" "BSA2 info"() -> (w1127:T23)
            n536 = global read "LDA_meas_global_1.vi" "BSA1 info"() -> (w1129:T23)
            n537 = Unbundle By Name(w1127) -> ("GPIB Address"=w1126:string)
            n538 = Unbundle By Name(w1129) -> ("GPIB Address"=w1128:string)
            n539 = call "Hydrosonic_Conrol.vi"("Input Mode"=enum16{"Desired Frequency", "Transducer value"}."Transducer value", "Desired Value"=w1130) -> ()  [unwired: 2 in, 2 out]
            n540 = call "Set_BSA_voltage_On_Off.vi"("GPIB address"=w1128, "High Voltage"=w1125) -> ()  [unwired: 1 in, 5 out]
            n541 = call "Set_BSA_voltage_On_Off.vi"("GPIB address"=w1126, "High Voltage"=w1125) -> ()  [unwired: 1 in, 5 out]
          }
        }
        n542 = case shown="True" w1095 {
          frame False {
          }
          frame True {
            n543 = global read "Preference_global.vi" "Rig Setup"() -> (w1114:string)
            n544 = Concatenate Strings(w1114, ":Program:Sync") -> (w1116:string)
            n545 = Bundle By Name(cluster=T19 {"Channel Name"="", "New Value"=0.0} ("Update Scan Value Cluster"), "Channel Name"=w1116, "New Value"=1000.0 ("Bundle Element")) -> (w1117:T19)
            n546 = Build Array(w1117) -> (w1119:T19[])
            n547 = call "Update_Current_Value_client.vi"("Update array in"=w1119) -> ()  [unwired: 1 in]
          }
        }
        n548 = Subtract(x=w1104, y=w1103) -> (x-y=w1102:dbl)
        n549 = Greater?(x=w1102, y=300.0) -> (0:w1099:bool)
        n550 = Not(x=w1099) -> (.not. x?=→"Non Starter":bool)
        n551 = Increment(x=w1089) -> (x+1=w1088:T3)
        n552 = Increment(x=w1088) -> (x+1=w1087:T3)
        n553 = Select(t=w1089, s=w1099, f=w1087) -> (s? t:f=w1100:T3)
      }
      frame "Email results to users" {
        n554 = local read "Currently on Row"() -> (w1137:i32)
        n555 = Increment(x=w1137) -> (x+1=w1132:i32)
        n556 = Split 1D Array(array=w1134, index=w1132) -> (first subarray=w1141:T6[], second subarray=w1140:T6[])
        n557 = Array Size(array=w1140) -> (size(s)=w1142:i32)
        n558 = for {
          tunnel: w1141 -> [w1157] mode=indexing
          shift-right: [w1155] -> w1143
          shift-left: string[] [] -> [w1156]
          n559 = Unbundle By Name(w1157) -> ("Row Type Selector"=w1148:T8, "Filename"=w1154:path, "Comments"=w1153:string)
          n560 = Not Equal?(x=Multi_run_mode."Auto Calibrate" ("Row Type Selector"), y=w1148) -> (x != y?=w1150:bool)
          n561 = Empty String/Path?(string/path=w1154) -> (empty?=w1151:bool)
          n562 = Compound Arithmetic op=AND(w1150, invert w1151) -> (w1149:bool)
          n563 = case shown="True" w1149 {
            tunnel: w1156 -> [w1158 w1166]
            tunnel: [w1158 w1165] -> w1155
            tunnel: w1154 -> [_ w1164]
            tunnel: w1153 -> [_ w1162]
            frame False {
            }
            frame True {
              n564 = Path To String(path=w1164) -> (string=w1163:string)
              n565 = Match Pattern(string=w1162, regular expression=" !!Program added comments") -> (after substring=w1159:string)  [unwired: 4 out]
              n566 = Concatenate Strings(w1163, w1159) -> (w1161:string)
              n567 = Build Array (concatenate)(w1166, w1161) -> (w1165:string[])
            }
          }
        }
        n568 = Equal To 0?(x=w1142) -> (x = 0?=w1133:bool)
        n569 = case shown="False" w1133 {
          tunnel: ["Having completed only some of the requested rows." ("Message") ""] -> w1138
          frame False {
          }
          frame True {
          }
        }
        n570 = call "End_of_run_messages.vi"("Message"=w1138, "Subject"="Multi Run Ended", "Attachments"=w1143) -> ()  [unwired: 1 in]
      }
      frame "Save run efficiency" {
        w1178 = FALSE  # append to file? (new file:F)
        w1177 = FALSE  # advisory dialog? (display:T)
        n571 = call "Setup_Filepath.vi"("Setup File Type"=Setup_Filetype."General", "Filename in"="Preferences.xls" ("name or relative path")) -> ("Filename Out"=w1167:path)  [unwired: 1 out]
        n572 = call "Overhead_Factor.vi"("Mode"=Overhead."Read Current Overhead") -> ("Current Overhead Factor"=w1172:dbl)  [unwired: 3 in]
        n573 = Number To Fractional String(number=w1172, precision (6)=i16 4) -> (F-format string=w1170:string)  [unwired: 2 out]
        n574 = call "Read_Characters_From_File.ph.vi"("file path (dialog if empty)"=w1167) -> ("character string"=w1175:string)  [unwired: 1 in, 7 out]
        n575 = call "Replace_data_in_setup_string.vi"("New data string"=w1170, "Input string"=w1175, "Variable name"="Current Overhead Factor") -> ("Appended string"=w1174:string)
        n576 = call "Write_Characters_To_File.vi"("file path (dialog if empty)"=w1167, "advisory dialog? (display:T)"=w1177, "character string"=w1174, "append to file? (new file:F)"=w1178) -> ()  [unwired: 1 in, 4 out]
      }
      frame "Remove Skipped Commands" {
        n577 = for {
          tunnel: w1184 -> [w1192] mode=indexing
          tunnel: [w1191] -> w1183 mode=indexing
          n578 = Unbundle By Name(w1192) -> ("Comments"=w1190:string)
          n579 = Match Pattern(string=w1190, regular expression=" !!Program added comments") -> (before substring=w1189:string)  [unwired: 4 out]
          n580 = Bundle By Name(cluster=w1192, "Comments"=w1189) -> (w1191:T6)
        }
      }
      frame "Show jumped positions" {
        n581 = global read "Trav_pos_global.vi" "Jumped Positions"() -> (w1195:dbl[][])
        n582 = Array Size(array=w1195) -> (size(s)=w1198:i32[])
        n583 = Index Array(array=w1198, index=0) -> (element=w1194:i32)
        n584 = Greater Than 0?(x=w1194) -> (x > 0?=w1196:bool)
        n585 = case shown="True" w1196 {
          tunnel: w1195 -> [_ w1209]
          tunnel: w1194 -> [_ w1208]
          frame False {
            w1202 = TRUE  # Front Panel Window:Is Frontmost
            n586 = Current VI's Path() -> (path=w1203:path)
            n587 = Open VI Reference(vi path=w1203) -> (vi reference=w1204:refnum<vi>, error out=w1205:errorcluster)  [unwired: 1 in, 4 out]
            n588 = property class="VI"(reference=w1204, error in=w1205, "Front Panel Window:Is Frontmost"=w1202) -> (reference out=w1206:refnum<vi>, error out=w1207:errorcluster)
            n589 = Close Reference(reference=w1206, error in (no error)=w1207) -> ()  [unwired: 1 out]
          }
          frame True {
            n590 = stacked-sequence {
              seq-local: [w1210 _ _] -> [_ w1222 _]
              tunnel: w1209 -> [w1211 _ w1231]
              tunnel: w1208 -> [_ w1225 _]
              frame #0 {
                n591 = local read "Work in Tunnel Coordinates?"() -> (w1212:T1)
                n592 = case shown="\"Work in Model Coordinates\"" w1212 {
                  tunnel: [w1214 w1220] -> w1210
                  tunnel: w1211 -> [w1213 w1220]
                  frame "Work in Tunnel Coordinates" {
                    n593 = global read "Trav_pos_global.vi" "Model Rotation (deg)"() -> (w1215:dbl)
                    n594 = for {
                      tunnel: w1215 -> [w1218]
                      tunnel: [w1217] -> w1214 mode=indexing
                      tunnel: w1213 -> [w1216] mode=indexing
                      n595 = call "Coordinate_rotation.vi"("Input Position"=w1216, "Coordinate rotation (deg)"=w1218, "Mode"=T21."To User Coordinates") -> ("Output Position"=w1217:dbl[])
                    }
                  }
                  frame "Work in Model Coordinates" {
                  }
                }
              }
              frame #1 {
                n596 = global read "Trav_pos_global.vi" "Default Traverse Setup"() -> (w1221:string)
                n597 = Format Into String(format string="There are %d points which cannot be reached", w1225) -> (resulting string=w1223:string)  [unwired: 2 in, 1 out]
                n598 = call "Display_Trav_Views.vi"("Current Probe Position"=w1222, "Traverse Name"=w1221, "Open Front Panel"=TRUE, "Error Comments"=w1223, "Crash?"=FALSE) -> ()  [unwired: 2 in, 4 out]
              }
              frame #2 {
                n599 = local read "Command filename"() -> (w1235:path)
                n600 = Array To Spreadsheet String(array=w1231, 3:"%.1f" ("format string")) -> (spreadsheet string=w1229:string)  [unwired: 1 out]
                n601 = Strip Path(path=w1235) -> (stripped path=w1234:path)  [unwired: 1 out]
                n602 = Build Path(base path=w1234, name or relative path="Jumped_Positions.xls") -> (appended path=w1232:path)
                n603 = call "Write_File_Simple.vi"("append to file? (new file:F)"=FALSE, "character string"=w1229, "file path"=w1232) -> ()  [unwired: 2 out]
              }
            }
          }
        }
      }
      frame "Save Setup to File" {
        w1252 = FALSE  # Start of Multi Run Prog
        n604 = Array Size(array=w1266) -> (size(s)=w1271:i32)
        n605 = local read "Last Row Run"() -> (w1241:i32)
        n606 = local read "Status"() -> (w1247:T2)
        n607 = local read "Stop after Repeats"() -> (w1250:bool)
        n608 = local read "stop"() -> (w1251:bool)
        n609 = Decrement(x=w1241) -> (x-1=w1242:i32)
        n610 = local read "Command filename"() -> (w1237:path)
        n611 = Increment(x=w1242) -> (x+1=w1254:i32)
        n612 = Equal?(x=w1247, y=Multi_Run_Status."Continue" ("Status")) -> (x = y?=w1246:bool)
        n613 = Compound Arithmetic op=OR(w1250, w1251, w1246) -> (w1249:bool)
        n614 = local read "Non Starter"() -> (w1259:bool)
        n615 = Select(t=w1254, s=w1249, f=w1242) -> (s? t:f=w1253:i32)
        n616 = Less?(x=w1245, y=T9."Run Multi Run Prog") -> (x < y?=w1243:bool)
        n617 = Equal?(x=w1271, y=w1241) -> (x = y?=w1261:bool)
        n618 = Equal To 0?(x=w1254) -> (x = 0?=w1260:bool)
        n619 = Split 1D Array(array=w1266, index=w1253) -> (second subarray=w1269:T6[])  [unwired: 1 out]
        n620 = Compound Arithmetic op=OR(w1261, w1260, w1259, w1243) -> (w1262:bool)
        n621 = call "Current_Filepath.vi"("Filename in"=w1237, "Data Type"="Commands") -> ("Filename Out"=w1236:path)  [unwired: 1 out]
        n622 = local read "Work in Tunnel Coordinates?"() -> (w1240:T1)
        n623 = local read "Jump Bad Positions"() -> (w1239:bool)
        n624 = case shown="False" w1262 {
          tunnel: w1236 -> [w1279 w1312]
          tunnel: [w1278 w1312] -> w1270
          tunnel: w1269 -> [w1276 _]
          tunnel: [w1275 w1313] -> w1268
          tunnel: w1266 -> [w1277 w1313]
          tunnel: w1240 -> [w1274 _]
          tunnel: w1239 -> [w1273 _]
          frame False {
            n625 = stacked-sequence {
              tunnel: w1279 -> [w1280 w1291 _]
              tunnel: [_ w1284 _] -> w1278
              tunnel: w1277 -> [w1283 _ w1296]
              tunnel: w1276 -> [_ _ w1294]
              tunnel: [_ _ w1293] -> w1275
              tunnel: w1274 -> [w1282 _ _]
              tunnel: w1273 -> [w1281 _ _]
              frame #0 {
                n626 = call "Save_Trav_setup.vi"("Work in Tunnel Coordinates?"=w1282, "Trav Table"=w1283, "Jump Bad Positions"=w1281, "Setup filename"=w1280) -> ()  [unwired: 2 out]
              }
              frame #1 {
                n627 = Strip Path(path=w1291) -> (stripped path=w1292:path, name=w1290:string)
                n628 = call "Add_filename_suffix.vi"("Filename"=w1290) -> ("Original Suffix"=w1287:string, "Base name"=w1289:string)  [unwired: 1 in, 2 out]
                n629 = Concatenate Strings(w1289, "_Rem", w1287) -> (w1286:string)
                n630 = Build Path(base path=w1292, name or relative path=w1286) -> (appended path=w1285:path)
                n631 = call "Find_Unique_Filename.vi"("Path In"=w1285) -> ("Unique Path Out"=w1284:path)  [unwired: 1 in, 1 out]
              }
              frame #2 {
                n632 = Index Array(array=w1296, index=0) -> (element=w1299:T6)
                n633 = Initialize Array(w1299, 0 ("dimension size")) -> (w1298:T6[])
                n634 = global read "Extra_Commands_Global.vi" "Minutes Before Repeating Row"() -> (w1297:string)
                n635 = for {
                  shift-right: [w1302] -> w1295
                  shift-left: w1298 -> [w1304]
                  tunnel: w1297 -> [w1306]
                  tunnel: w1296 -> [w1303] mode=indexing
                  n636 = Unbundle By Name(w1303) -> ("Extra Commands"=w1305:string)
                  n637 = call "Extra_Commands.vi"("String to Search"=w1305, "Command"=w1306) -> ("Command Found"=w1307:bool)  [unwired: 1 in, 4 out]
                  n638 = case shown="False" w1307 {
                    tunnel: w1304 -> [w1308 w1311]
                    tunnel: w1303 -> [_ w1310]
                    tunnel: [w1308 w1309] -> w1302
                    frame False {
                    }
                    frame True {
                      n639 = Build Array (concatenate)(w1311, w1310) -> (w1309:T6[])
                    }
                  }
                }
                n640 = Build Array (concatenate)(w1295, w1294) -> (w1293:T6[])
              }
            }
          }
          frame True {
          }
        }
        n641 = Path To String(path=w1236) -> (string=w1258:string)
        n642 = Concatenate Strings("Multi run Prog Ended having the setup filename of :" ("Message"), w1258) -> (w1257:string)
        n643 = call "Save_Trav_setup.vi"("Work in Tunnel Coordinates?"=w1240, "Trav Table"=w1268, "Jump Bad Positions"=w1239, "Setup filename"=w1270) -> ("Trav Table Out"=w1267:T6[])  [unwired: 1 out]
        n644 = call "Log_Current_row_to_Execute.vi"("Simulate/Run"=w1256, "Message"=w1257, "Start of Multi Run Prog"=w1252) -> ()  [unwired: 2 in, 5 out]
        n645 = Select(t=w1267, s=w1262, f=w1266) -> (s? t:f=w1265:T6[])
      }
      frame "End" {
        w1315 = ""
        w1317 = path ""
        w1318 = 0 ("No. of pts.")
        w1320 = nan
        n646 = global write "Trav_pos_global.vi" "Top level setup filename"(w1317) -> ()
        n647 = global read "Trav_pos_global.vi" "Current Row"() -> (w1324:T6)
        n648 = Bundle By Name(cluster=w1324, "Start X"=w1320, "Start Y"=w1320, "Start Z"=w1320, "End X"=w1320, "End Y"=w1320, "End Z"=w1320, "No. of pts."=w1318, "Spacing"=Spacing."Linear", "Filename"=w1317, "Tunnel Speed"=w1320, "Averaging time (min)"=w1320, "Extra Commands"=w1315, "Specific Arguments"=w1315, "Emission Rate (l/min)"=w1320, "Trace Gas Concentration (%)"=w1320, "Density Ratio"=w1315, "Comments"=w1315, "Row No"=w1318, "Row Type Selector"=Multi_run_mode."Blank Row", "Completion time"=w1315, "Meas Setup File"=w1315, "Row Duration (mins)"=w1320, "No. of Valid pts."=w1318) -> (w1323:T6)
        n649 = Current VI's Path() -> (path=w1316:path)
        n650 = global write "Trav_pos_global.vi" "Current Row"(w1323) -> ()
        n651 = global write "Trav_pos_global.vi" "Meas Setup Number"(0 ("Meas Setup Number")) -> ()
        n652 = call "Bring_to_front.vi"("path"=w1316) -> ()
        n653 = global write "Trav_pos_global.vi" "Estimated Completion time"("") -> ()
        n654 = Build Array(u32 0) -> (w1325:u32[])
        n655 = property on="Table" class="Arr (strict)"("Index Values"=w1325) -> ()  [unwired: 2 in, 2 out]
      }
    }
    n656 = case shown="False" w8 {
      tunnel: w4 -> [_ w15]
      frame False {
      }
      frame True {
        n657 = local write "Table"(w15) -> ()
      }
    }
    "Multi Run Case" <- w10
  }
